vi "TPM and WF version 8-3.vi"() -> ()   [LabVIEW 2012]
uses:
  <vilib>/_Imagine Optic/VIs drivers/Data Haso/Wavefront parameters.ctl
  <vilib>/Utility/error.llb/DialogType.ctl
  Program Files/Imagine Optic/Casao LabVIEW SDK/Casao/Casao/Loop prefs.ctl
  <vilib>/_Imagine Optic/VIs drivers/Data Haso/DataHaso.ctl
  <vilib>/DAQmx/write.llb/DAQmx Write (Digital Bool 1Line 1Point).vi
  <vilib>/DAQmx/write.llb/DAQmx Write (Analog DBL 1Chan 1Samp).vi
  <vilib>/DAQmx/write.llb/DAQmx Write (Analog 1D Wfm NChan NSamp).vi
  <vilib>/DAQmx/create/channels.llb/DAQmx Create Channel (DO-Digital Output).vi
  <vilib>/DAQmx/create/channels.llb/DAQmx Create Channel (AO-Voltage-Basic).vi
  <vilib>/DAQmx/miscellaneous.llb/DAQmx Fill In Error Info.vi
  <vilib>/Analysis/coordinate.llb/2D Cartesian Coordinate Rotation (Array).vi
  <vilib>/DAQmx/configure/timing.llb/DAQmx Timing (Use Waveform).vi
  <vilib>/DAQmx/configure/trigger.llb/DAQmx Start Trigger (Digital Edge).vi
  <vilib>/measure/NI_MABase.lvlib
  <vilib>/Analysis/NI_AALPro.lvlib
panel:
  in  "Tab Control":enum32{"TPM imaging", "Wavefront sensor"}(tab)
  in  "Boolean 3":bool
  in  "Y offset (Pixel)":dbl=501.0
  in  "X offset (pixel)":dbl=502.0
  in  "Area Scale factor(0-1)":dbl=1.0
  in  "Model":i16(ring)=-5 items=["Phase"=1, "Imaging"=-5]
  out "Boolean":bool
  in  "Pockel Cell Correction Phase":dbl=135.0
  in  "Repeat time":dbl=100.0
  in  "Laser power %(0-100)":dbl=10.0
  in  "Exp Time":u32(ring)=500000 items=["0.5s"=500000, "1.0s"=1000000, "1.5s"=1500000]
  out "RMS 2":dbl
  out "PV 2":dbl
  in  "Filter x tilt 2":bool=TRUE
  in  "Filter y tilt 2":bool=TRUE
  in  "Curvature filter 2":bool=TRUE
  out "after correction":T1
  in  "Boolean 2":bool
  out "after correction":dbl[][](graph) caption="Wavefront"
  out "before correction":dbl[][](graph) caption="Wavefront"
  in  "Matrix path":path=path "C:/Documents and Settings/User/Desktop/zw/20160103 interaction matrix 1um bead step0.2.aomc"
  in  "Phase modulator config file path":path=path "C:/Program Files/Imagine Optic/Configuration Files/mirao 52-e 0225.xml"
  in  "Haso serial number":u32=7364
  in  "Scale factor":u16=1
  in  "Power%(0-100)":dbl=10.0
  in  "Filter x tilt":bool=TRUE
  in  "Filter y tilt":bool=TRUE
  in  "Curvature filter":bool=TRUE
  out "Parameters":T1
  out "Camera image":u32[][](graph)
  out "PV":dbl
  out "RMS":dbl
  # "For small area setting"
  # "Measure"
  # "Correction"
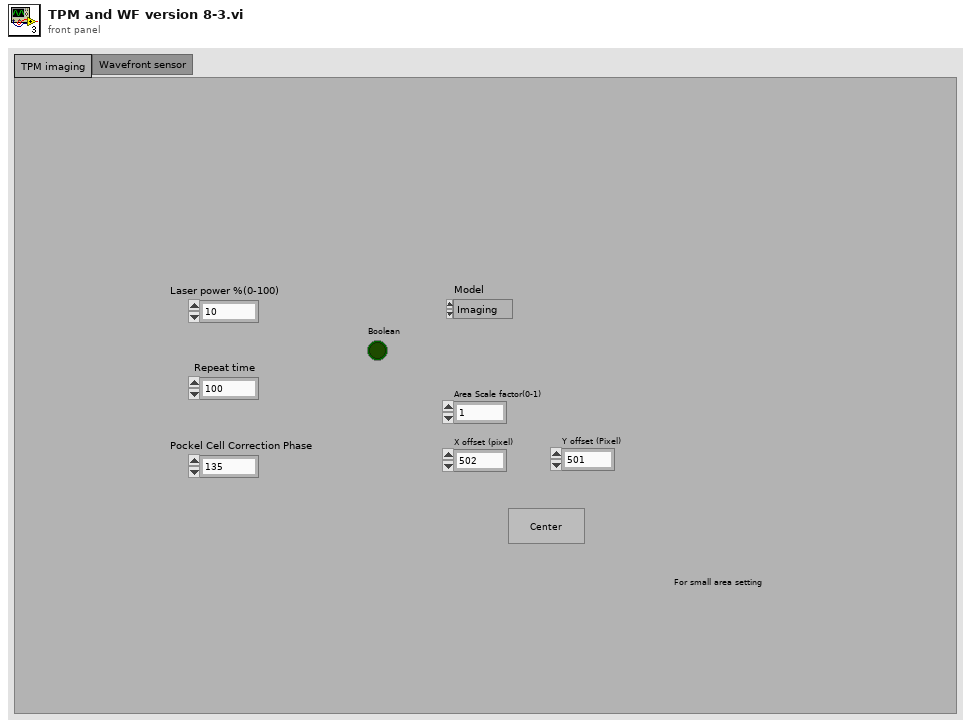
[diagram p1: front panel]
types:
  T1 = typedef "Wavefront parameters.ctl" = cluster{"X Tilt (mrad)":sgl, "Y Tilt (mrad)":sgl, "Radius of curvature (mm)":sgl, "X focal point position (mm)":sgl, "Y focal point position (mm)":sgl, "Astigmatism angle (rad)":sgl, "Sagittal focal length (mm)":sgl, "Tangential focal length (mm)":sgl}
  T2 = cluster{"Galvo/Pockels Cell Sampling Info":dbl, "#s":dbl}
  T3 = cluster{"Filtre tilt X":bool, "Filtre tilt Y":bool, "Filtre courbure":bool}
  T4 = typedef "Loop prefs.ctl" = cluster{"Filter tilt on measurement (closed loop)":bool, "Correction gain (closed loop)":sgl, "Limit of subapertures off in CGP (%)":sgl, "Limit of saturated actuators (%)":sgl}
  T5 = typedef "DataHaso.ctl" = i32
  T6 = cluster{"Measurement":T5, "Target":T5, "Manual target":T5}
  T7 = cluster{"Target for tilt":T5, "Target for focus":T5, "Target for all other aberrations":T5}
  T8 = typedef "DialogType.ctl" = u16
  T9 = typedef "Haso.ctl" = i32
  T10 = typedef "Camera.ctl" = i32
  T11 = typedef "Camera preferences.ctl" = cluster{"Exposure duration (µs)":u32, "Exposure duration specified (µs)":u32, "Number of summed images":u32, "Trigger type":enum16{"Internal", "TTL", "Software"}, "Trigger event":enum16{"falling", "rising"}, "Remove background image":bool, "Background image":T12, "Path to background image":string, "Auto exposure":bool, "Auto exposure target (%)":sgl, "Auto exposure tolerance (%)":sgl, "Timeout delay (ms)":u32, "Delay after trigger (µs)":i32}
  T12 = typedef "Image Compat.ctl" = cluster{"Signed/unsigned":bool, "Number of bits":T13, "Internal object id":i32, "Internal data id":i32}
  T13 = typedef "Data alignment enum.ctl" = enum16{"8", "16", "32"}
  T14 = typedef "Casao.ctl" = i32
  T15 = typedef "CasaoMatrix.ctl" = i32
  T16 = typedef "PhaseModul.ctl" = i32
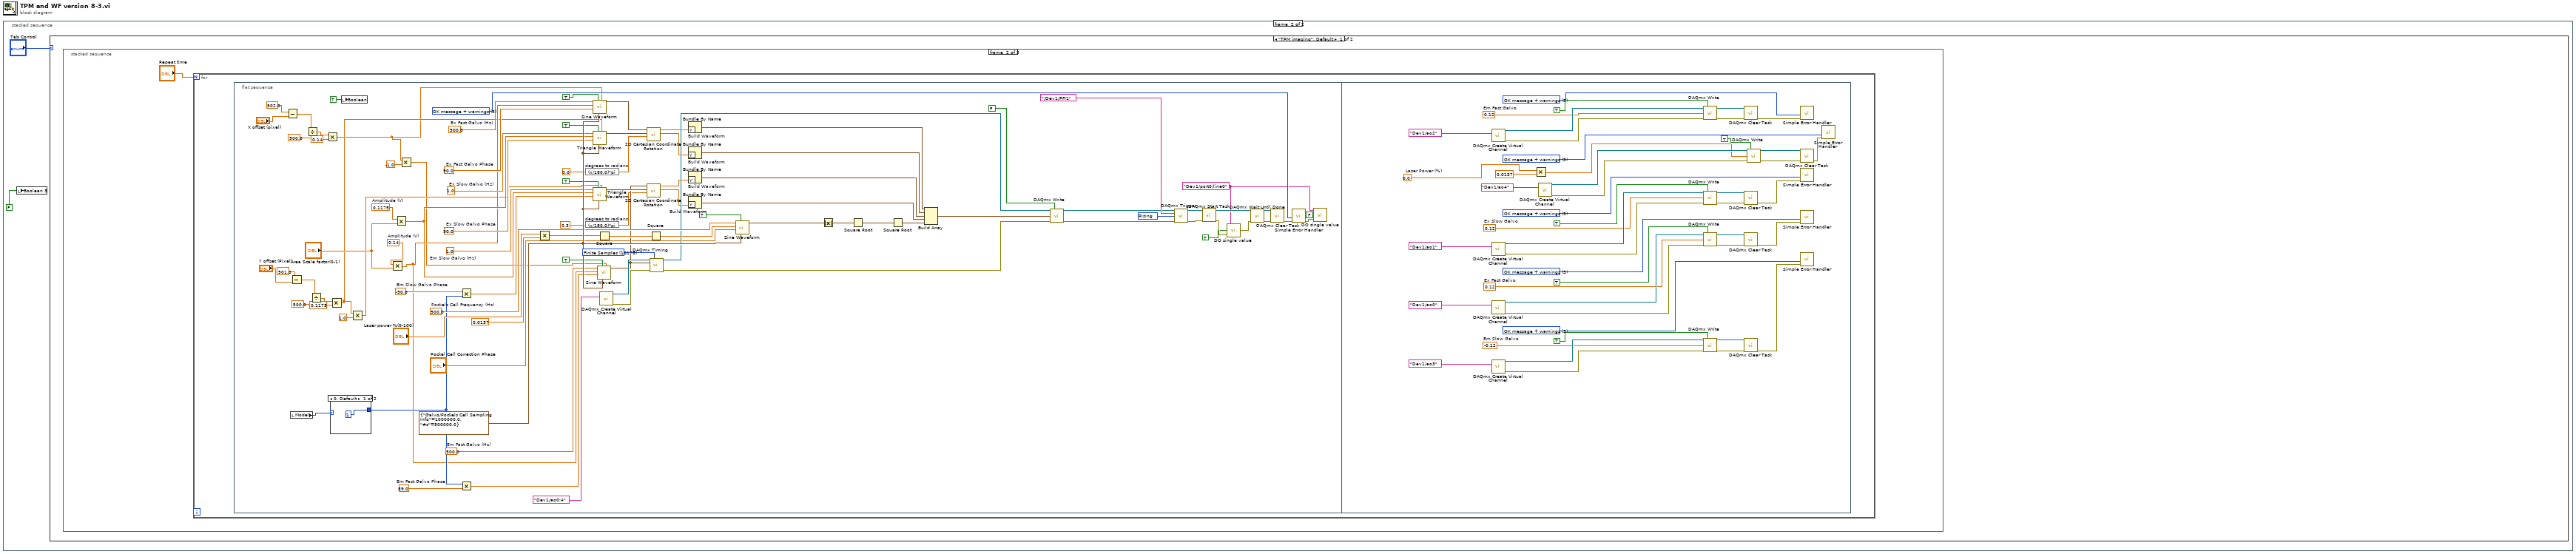
[diagram p0: block diagram]
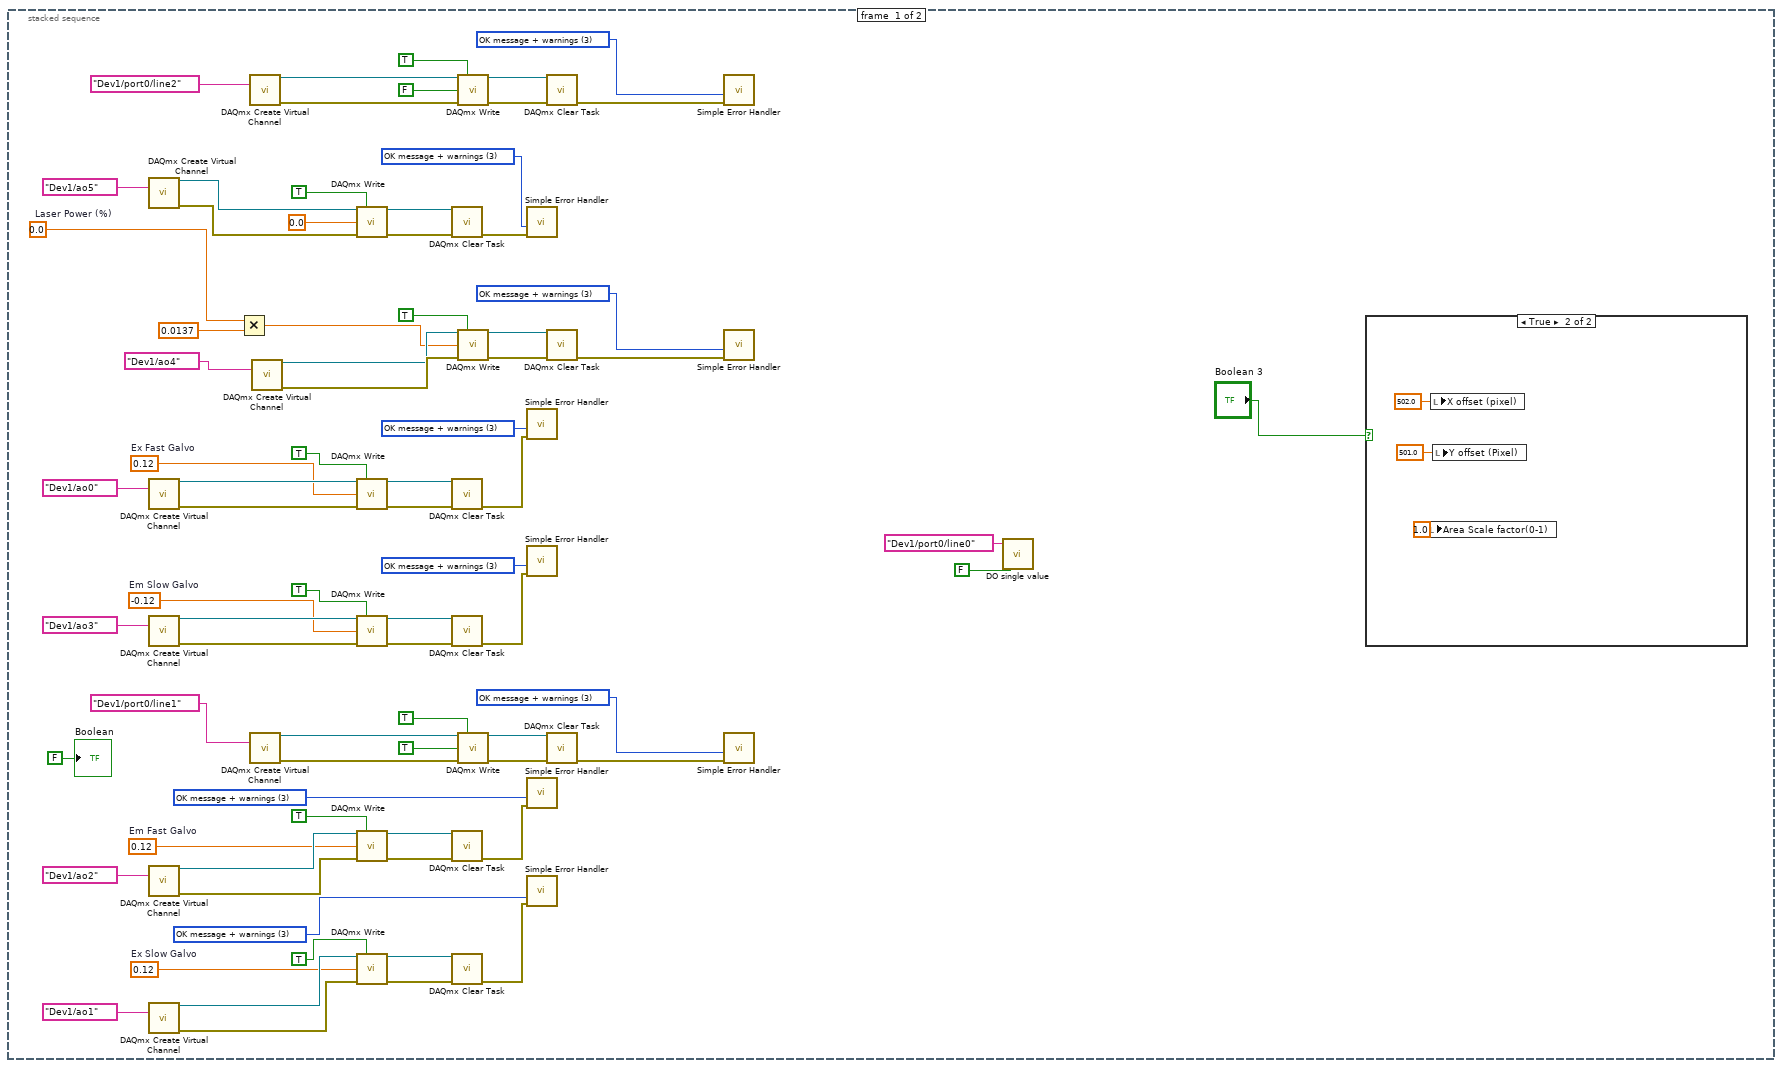
[diagram p2: hidden frame]
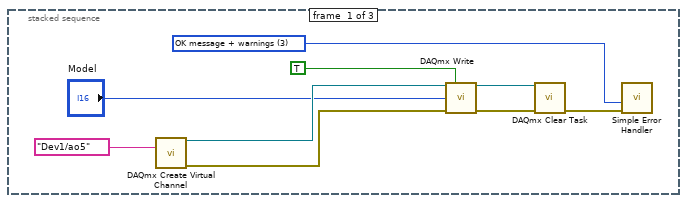
[diagram p4: hidden frame]
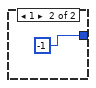
[diagram p5: hidden frame]
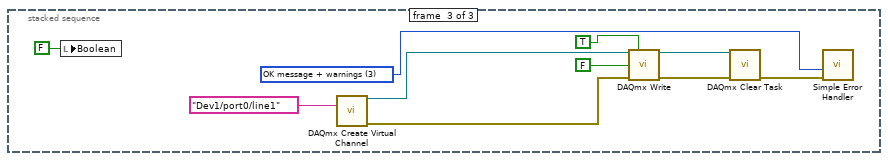
[diagram p6: hidden frame]
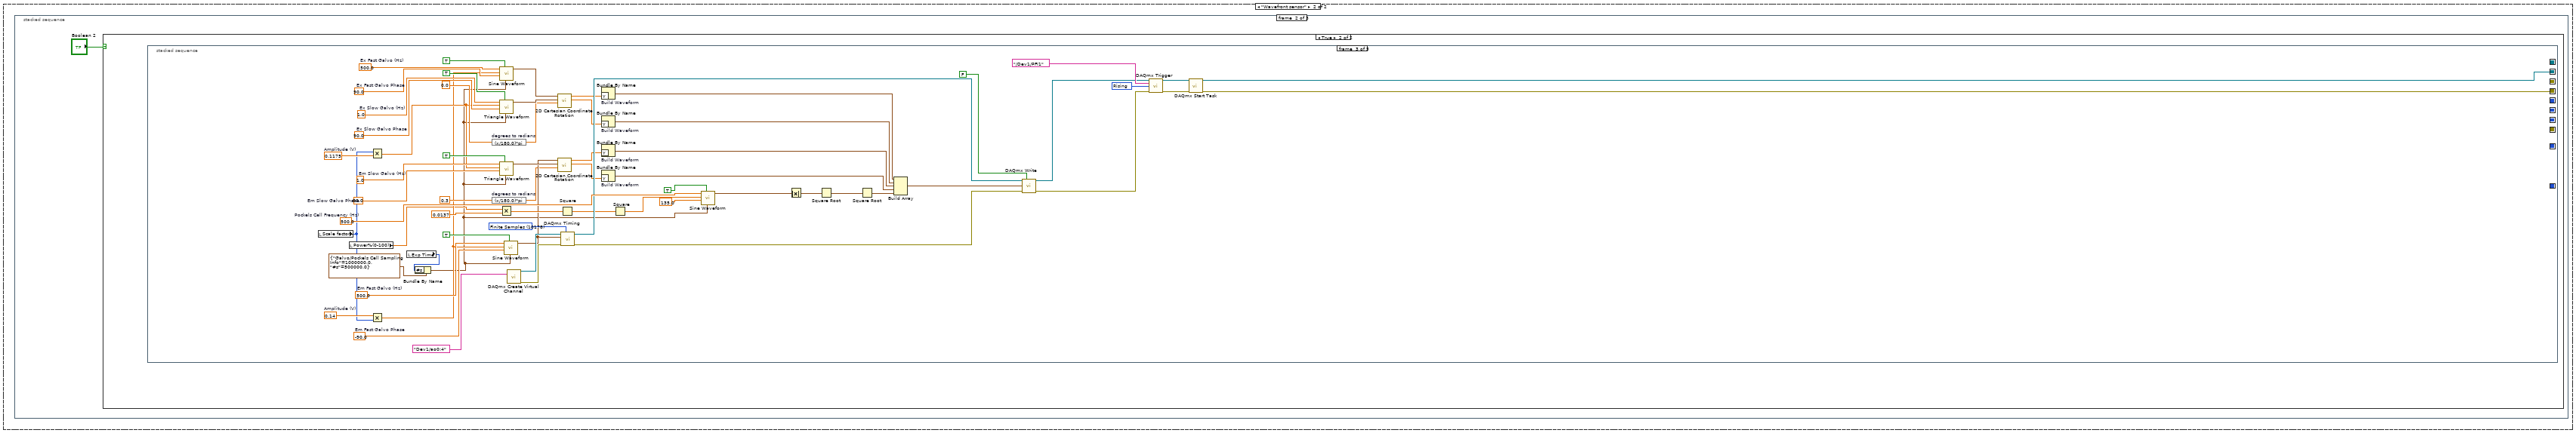
[diagram p7: hidden frame]
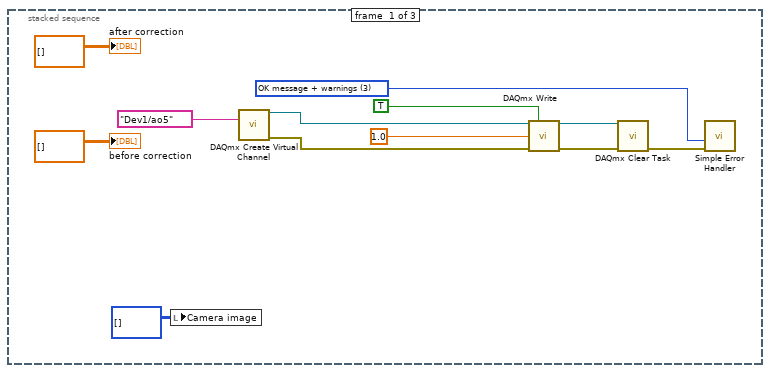
[diagram p8: hidden frame]
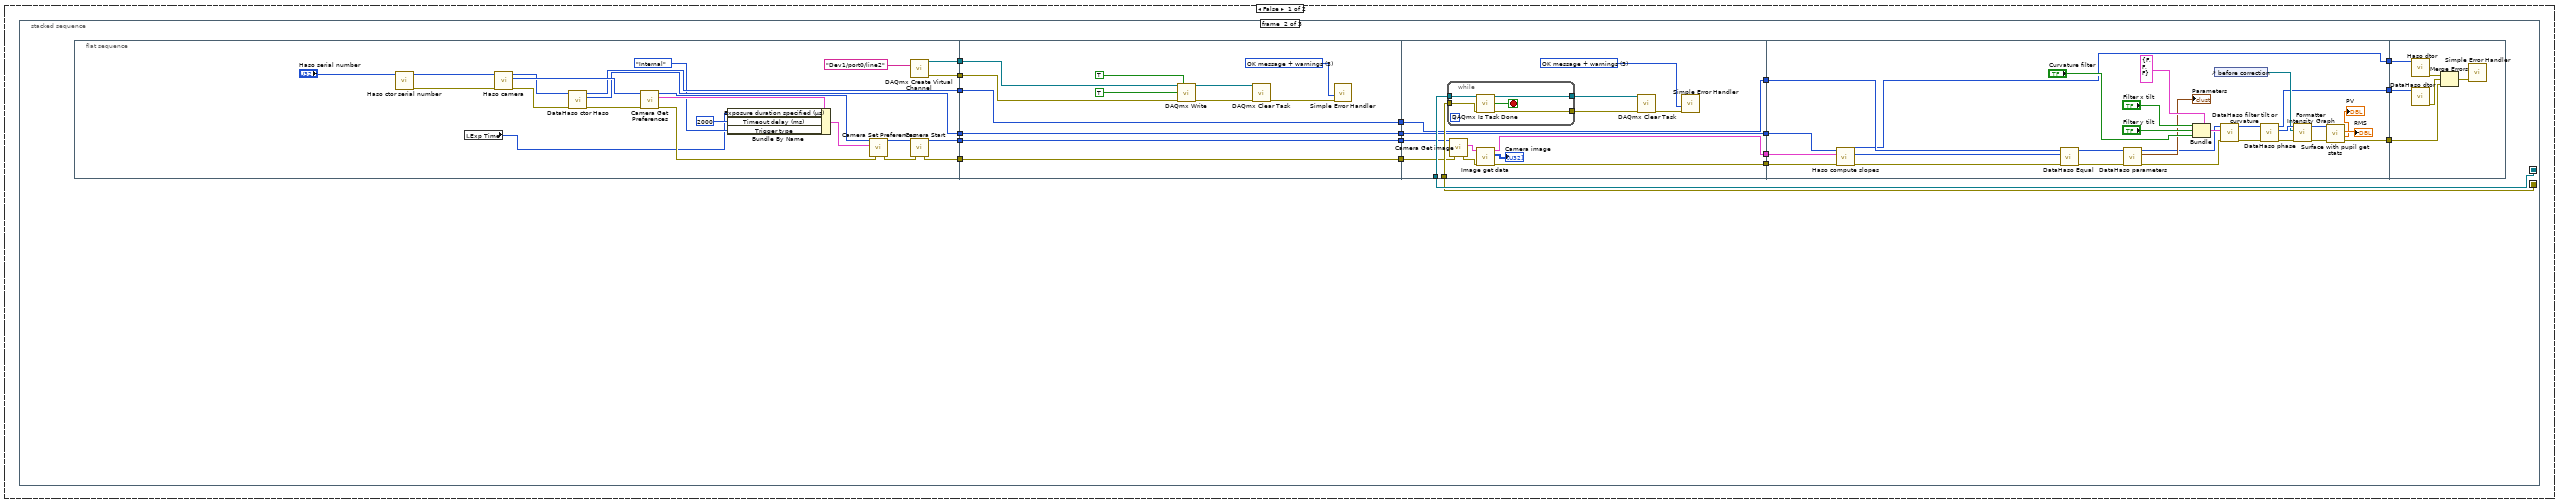
[diagram p9: hidden frame]
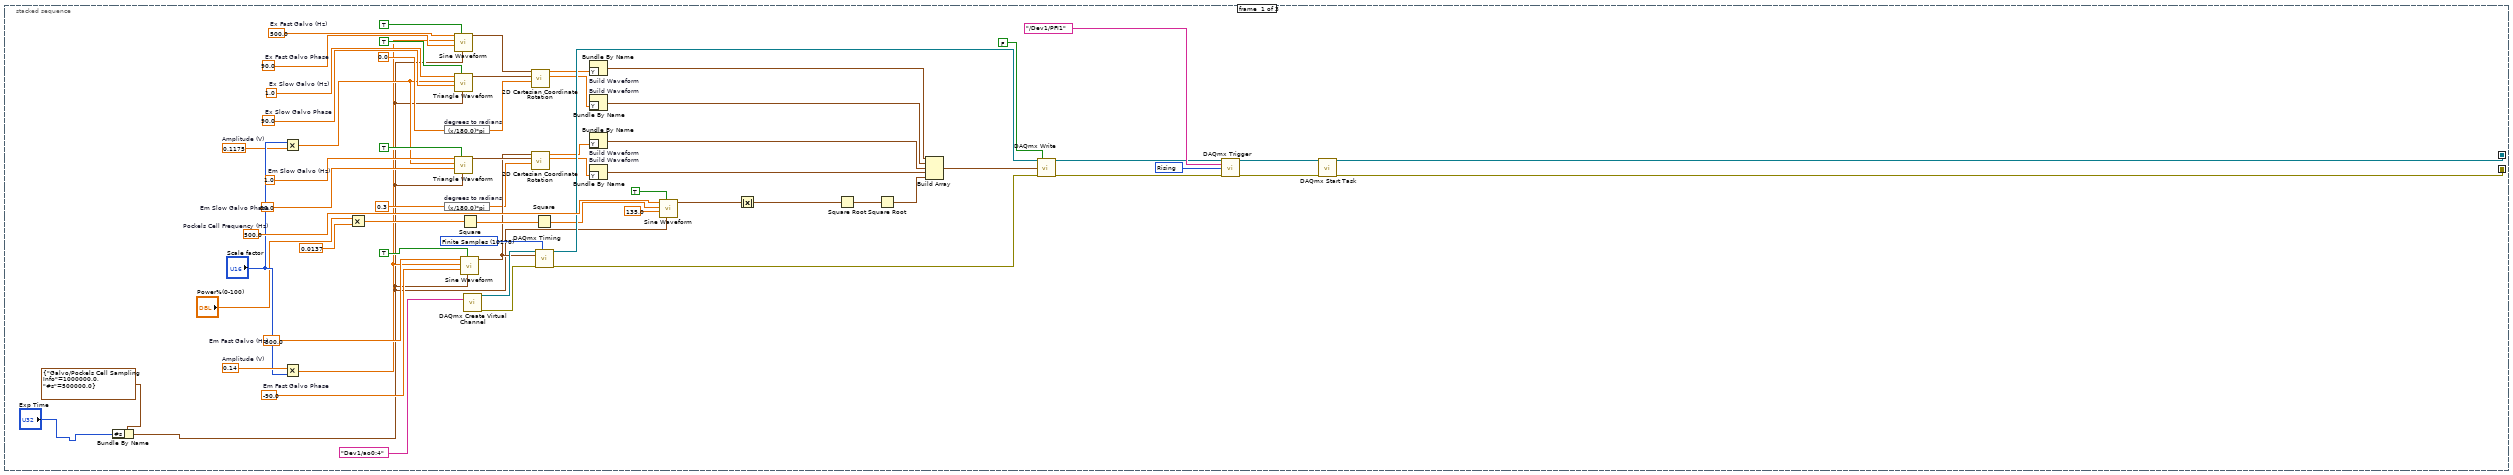
[diagram p10: hidden frame]
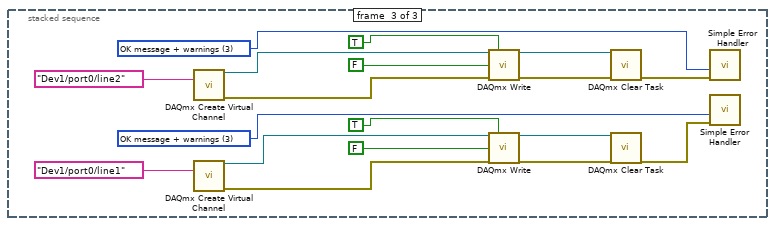
[diagram p11: hidden frame]
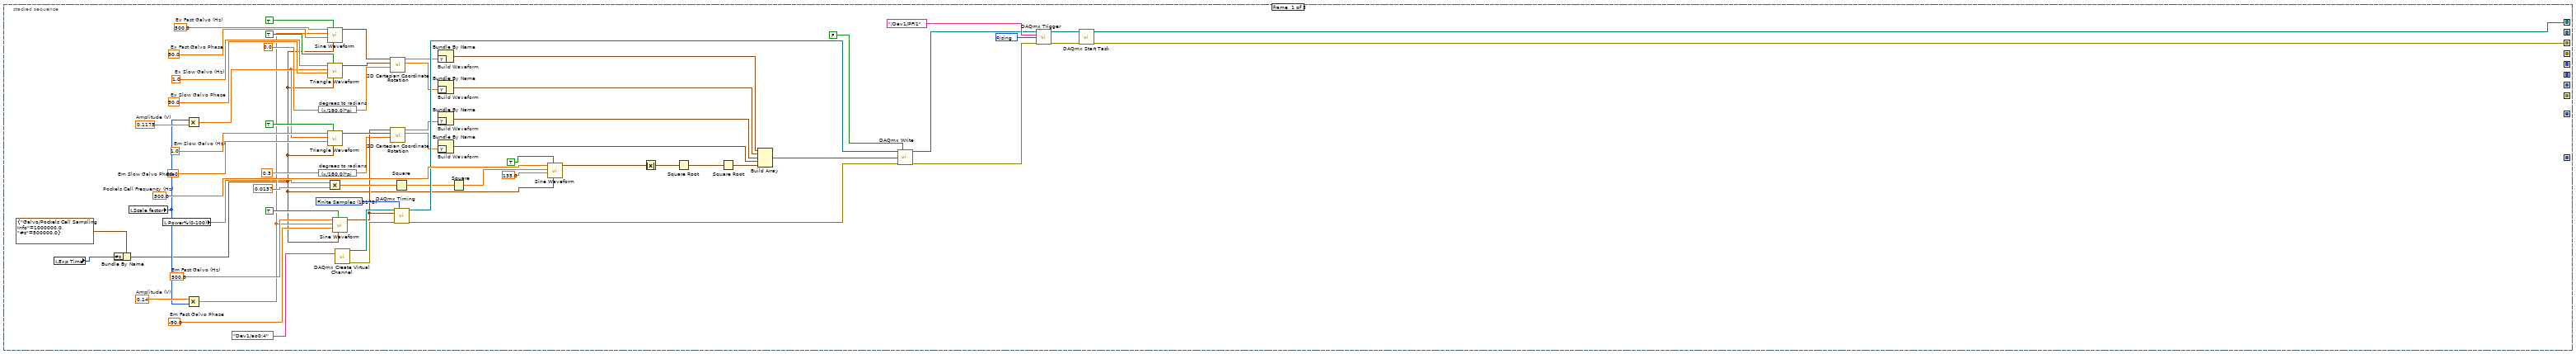
[diagram p12: hidden frame]
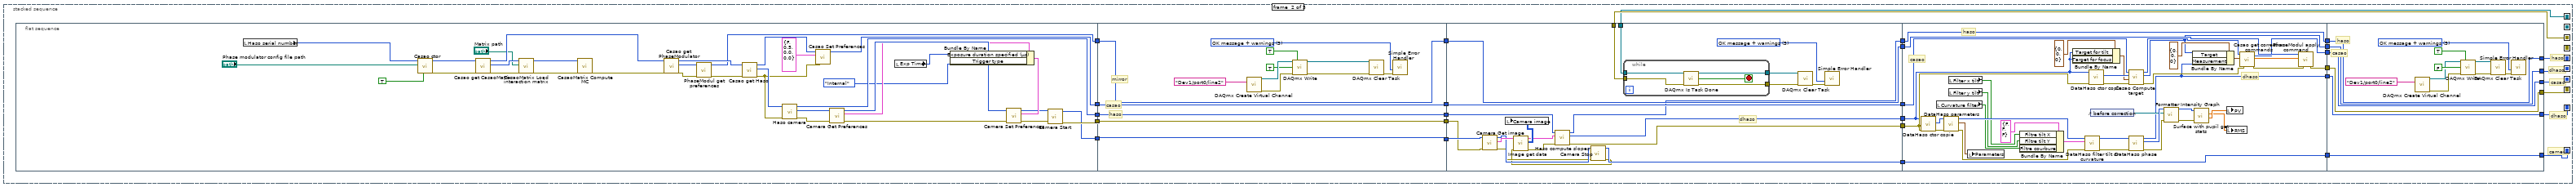
[diagram p13: hidden frame]
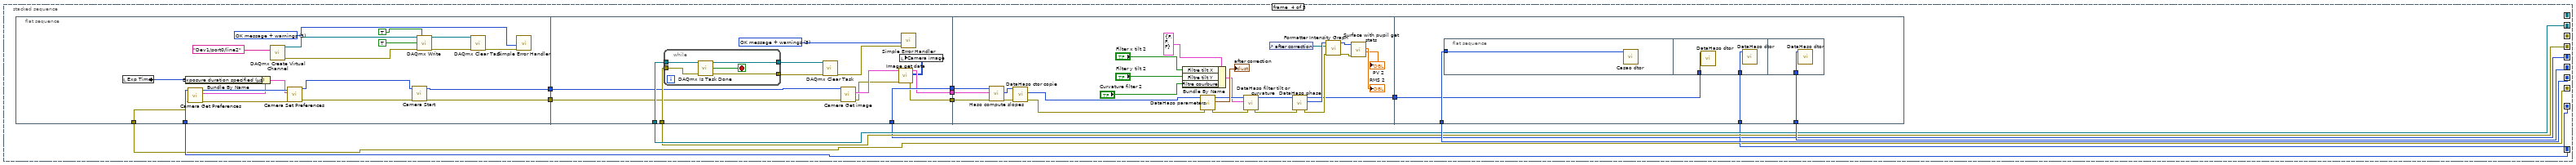
[diagram p14: hidden frame]
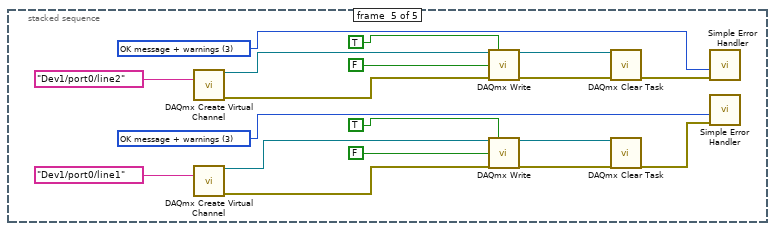
[diagram p15: hidden frame]
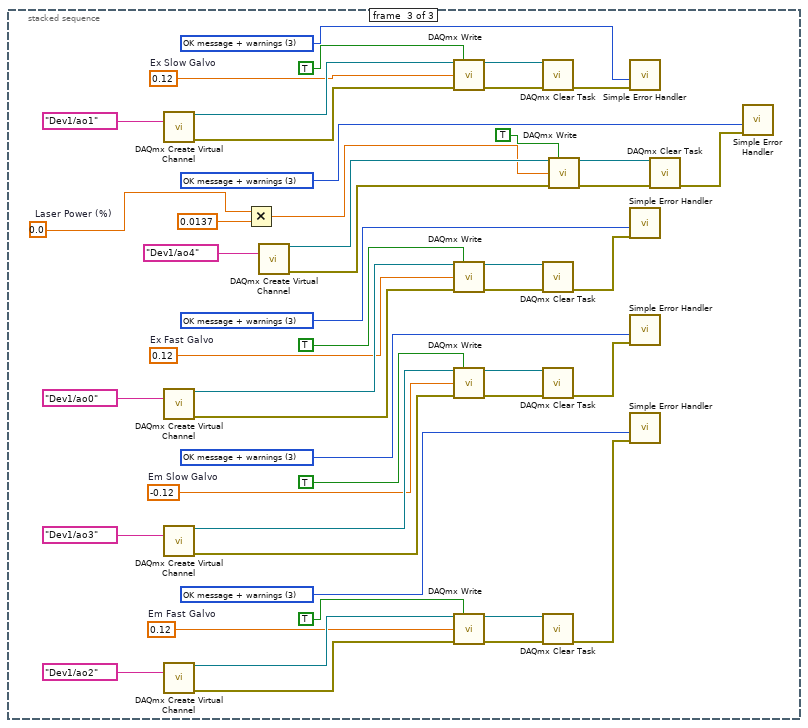
[diagram p16: hidden frame]
diagram:
  n1 = stacked-sequence {
    frame #0 {
      w11 = T8 3 items=["no dialog", "OK message", "continue or stop message", "OK message + warnings", "continue/stop + warnings"] ("type of dialog (OK msg:1)")
      w20 = T8 3 items=["no dialog", "OK message", "continue or stop message", "OK message + warnings", "continue/stop + warnings"] ("type of dialog (OK msg:1)")
      w59 = 0.0  # Laser Power (%)
      w41 = 0.12  # Em Fast Galvo
      w23 = -0.12  # Em Slow Galvo
      w32 = 0.12  # Ex Slow Galvo
      w50 = 0.12  # Ex Fast Galvo
      w29 = T8 3 items=["no dialog", "OK message", "continue or stop message", "OK message + warnings", "continue/stop + warnings"] ("type of dialog (OK msg:1)")
      w38 = T8 3 items=["no dialog", "OK message", "continue or stop message", "OK message + warnings", "continue/stop + warnings"] ("type of dialog (OK msg:1)")
      w47 = T8 3 items=["no dialog", "OK message", "continue or stop message", "OK message + warnings", "continue/stop + warnings"] ("type of dialog (OK msg:1)")
      w56 = T8 3 items=["no dialog", "OK message", "continue or stop message", "OK message + warnings", "continue/stop + warnings"] ("type of dialog (OK msg:1)")
      w62 = T8 3 items=["no dialog", "OK message", "continue or stop message", "OK message + warnings", "continue/stop + warnings"] ("type of dialog (OK msg:1)")
      w77 = T8 3 items=["no dialog", "OK message", "continue or stop message", "OK message + warnings", "continue/stop + warnings"] ("type of dialog (OK msg:1)")
      n2 = call-poly <vilib>:"DAQmx Create Virtual Channel.vi"("physical channels"=tag "Dev1/ao5") -> ("task out"=w16:refnum<k21>, "error out"=w15:errorcluster)  [unwired: 13 in]
      n3 = call-poly <vilib>:"DAQmx Create Virtual Channel.vi"("physical channels"=tag "Dev1/ao0") -> ("task out"=w52:refnum<k21>, "error out"=w51:errorcluster)  [unwired: 13 in]
      n4 = call-poly <vilib>:"DAQmx Create Virtual Channel.vi"("physical channels"=tag "Dev1/ao3") -> ("task out"=w25:refnum<k21>, "error out"=w24:errorcluster)  [unwired: 13 in]
      n5 = call-poly <vilib>:"DAQmx Create Virtual Channel.vi"("physical channels"=tag "Dev1/ao2") -> ("task out"=w43:refnum<k21>, "error out"=w42:errorcluster)  [unwired: 13 in]
      n6 = call-poly <vilib>:"DAQmx Create Virtual Channel.vi"("physical channels"=tag "Dev1/ao1") -> ("task out"=w34:refnum<k21>, "error out"=w33:errorcluster)  [unwired: 13 in]
      n7 = Multiply(x=w59, y=0.0137 ("data")) -> (x*y=w61:dbl)
      n8 = call-poly <vilib>:"DAQmx Create Virtual Channel.vi"("lines"=tag "Dev1/port0/line2") -> ("task out"=w7:refnum<k21>, "error out"=w8:errorcluster)  [unwired: 13 in]
      n9 = call-poly <vilib>:"DAQmx Create Virtual Channel.vi"("lines"=tag "Dev1/port0/line1") -> ("task out"=w73:refnum<k21>, "error out"=w74:errorcluster)  [unwired: 13 in]
      n10 = call-poly <vilib>:"DAQmx Create Virtual Channel.vi"("physical channels"=tag "Dev1/ao4") -> ("task out"=w68:refnum<k21>, "error out"=w69:errorcluster)  [unwired: 13 in]
      n11 = call-poly <vilib>:"DAQmx Write.vi"("task/channels in"=w16, "auto start"=TRUE, "data"=0.0, "error in"=w15) -> ("task out"=w18:refnum<k21>, "error out"=w17:errorcluster)  [unwired: 9 in, 1 out]
      n12 = call-poly <vilib>:"DAQmx Write.vi"("task/channels in"=w52, "auto start"=TRUE, "data"=w50, "error in"=w51) -> ("task out"=w54:refnum<k21>, "error out"=w53:errorcluster)  [unwired: 9 in, 1 out]
      n13 = call-poly <vilib>:"DAQmx Write.vi"("task/channels in"=w25, "auto start"=TRUE, "data"=w23, "error in"=w24) -> ("task out"=w27:refnum<k21>, "error out"=w26:errorcluster)  [unwired: 9 in, 1 out]
      n14 = call-poly <vilib>:"DAQmx Write.vi"("task/channels in"=w43, "auto start"=TRUE, "data"=w41, "error in"=w42) -> ("task out"=w45:refnum<k21>, "error out"=w44:errorcluster)  [unwired: 9 in, 1 out]
      n15 = call-poly <vilib>:"DAQmx Write.vi"("task/channels in"=w34, "auto start"=TRUE, "data"=w32, "error in"=w33) -> ("task out"=w36:refnum<k21>, "error out"=w35:errorcluster)  [unwired: 9 in, 1 out]
      n16 = call <vilib>:"DAQmx Clear Task.vi"("task in"=w18, "error in"=w17) -> ("error out"=w19:errorcluster)  [unwired: 13 in]
      n17 = call <vilib>:"DAQmx Clear Task.vi"("task in"=w54, "error in"=w53) -> ("error out"=w55:errorcluster)  [unwired: 13 in]
      n18 = call <vilib>:"DAQmx Clear Task.vi"("task in"=w27, "error in"=w26) -> ("error out"=w28:errorcluster)  [unwired: 13 in]
      n19 = call <vilib>:"DAQmx Clear Task.vi"("task in"=w45, "error in"=w44) -> ("error out"=w46:errorcluster)  [unwired: 13 in]
      n20 = call <vilib>:"DAQmx Clear Task.vi"("task in"=w36, "error in"=w35) -> ("error out"=w37:errorcluster)  [unwired: 13 in]
      n21 = call-poly <vilib>:"DAQmx Write.vi"("task/channels in"=w7, "auto start"=TRUE, "data"=FALSE ("Shutter"), "error in"=w8) -> ("task out"=w5:refnum<k21>, "error out"=w4:errorcluster)  [unwired: 9 in, 1 out]
      n22 = call-poly <vilib>:"DAQmx Write.vi"("task/channels in"=w68, "auto start"=TRUE, "data"=w61, "error in"=w69) -> ("task out"=w65:refnum<k21>, "error out"=w66:errorcluster)  [unwired: 9 in, 1 out]
      n23 = call-poly <vilib>:"DAQmx Write.vi"("task/channels in"=w73, "auto start"=TRUE, "data"=TRUE ("Shutter"), "error in"=w74) -> ("task out"=w71:refnum<k21>, "error out"=w70:errorcluster)  [unwired: 9 in, 1 out]
      n24 = call <vilib>:"Simple Error Handler.vi"("type of dialog (OK msg:1)"=w20, "error in (no error)"=w19) -> ()  [unwired: 3 in, 5 out]
      n25 = call <vilib>:"Simple Error Handler.vi"("type of dialog (OK msg:1)"=w56, "error in (no error)"=w55) -> ()  [unwired: 3 in, 5 out]
      n26 = call <vilib>:"Simple Error Handler.vi"("type of dialog (OK msg:1)"=w29, "error in (no error)"=w28) -> ()  [unwired: 3 in, 5 out]
      n27 = call <vilib>:"Simple Error Handler.vi"("type of dialog (OK msg:1)"=w47, "error in (no error)"=w46) -> ()  [unwired: 3 in, 5 out]
      n28 = call <vilib>:"Simple Error Handler.vi"("type of dialog (OK msg:1)"=w38, "error in (no error)"=w37) -> ()  [unwired: 3 in, 5 out]
      n29 = call <vilib>:"DAQmx Clear Task.vi"("task in"=w5, "error in"=w4) -> ("error out"=w10:errorcluster)  [unwired: 13 in]
      n30 = call <vilib>:"DAQmx Clear Task.vi"("task in"=w65, "error in"=w66) -> ("error out"=w63:errorcluster)  [unwired: 13 in]
      n31 = call <vilib>:"DAQmx Clear Task.vi"("task in"=w71, "error in"=w70) -> ("error out"=w76:errorcluster)  [unwired: 13 in]
      n32 = call <vilib>:"Simple Error Handler.vi"("type of dialog (OK msg:1)"=w11, "error in (no error)"=w10) -> ()  [unwired: 3 in, 5 out]
      n33 = call <vilib>:"Simple Error Handler.vi"("type of dialog (OK msg:1)"=w62, "error in (no error)"=w63) -> ()  [unwired: 3 in, 5 out]
      n34 = call <vilib>:"Simple Error Handler.vi"("type of dialog (OK msg:1)"=w77, "error in (no error)"=w76) -> ()  [unwired: 3 in, 5 out]
      n35 = call "DO single value.vi"("data"=FALSE, "lines"=tag "Dev1/port0/line0") -> ()  [unwired: 1 in, 1 out]
      n36 = case shown="True" "Boolean 3" {
        frame False {
        }
        frame True {
          n37 = local write "Area Scale factor(0-1)"(1.0 ("Scale factor(0-1)")) -> ()
          n38 = local write "X offset (pixel)"(502.0 ("X offset (pixel)")) -> ()
          n39 = local write "Y offset (Pixel)"(501.0 ("Y offset (Pixel)")) -> ()
        }
      }
      "Boolean" <- FALSE ("Boolean")
    }
    frame #1 {
      n40 = local write "Boolean 3"(FALSE ("Boolean 3")) -> ()
      n41 = case shown="\"TPM imaging\", Default" "Tab Control" {
        frame "TPM imaging", Default {
          n42 = stacked-sequence {
            frame #0 {
              w87 = T8 3 items=["no dialog", "OK message", "continue or stop message", "OK message + warnings", "continue/stop + warnings"] ("type of dialog (OK msg:1)")
              n43 = call-poly <vilib>:"DAQmx Create Virtual Channel.vi"("physical channels"=tag "Dev1/ao5") -> ("task out"=w91:refnum<k21>, "error out"=w92:errorcluster)  [unwired: 13 in]
              n44 = call-poly <vilib>:"DAQmx Write.vi"("task/channels in"=w91, "auto start"=TRUE, "data"="Model", "error in"=w92) -> ("task out"=w89:refnum<k21>, "error out"=w90:errorcluster)  [unwired: 9 in, 1 out]
              n45 = call <vilib>:"DAQmx Clear Task.vi"("task in"=w89, "error in"=w90) -> ("error out"=w88:errorcluster)  [unwired: 13 in]
              n46 = call <vilib>:"Simple Error Handler.vi"("type of dialog (OK msg:1)"=w87, "error in (no error)"=w88) -> ()  [unwired: 3 in, 5 out]
            }
            frame #1 {
              n47 = for {
                N: "Repeat time" -> [_]
                n48 = flat-sequence {
                  frame #0 {
                    w118 = tag "Dev1/port0/line0" ("lines")
                    w129 = 89.0  # Em Fast Galvo Phase
                    w186 = 1.0  # Em Slow Galvo (Hz)
                    w184 = 1.0  # Ex Slow Galvo (Hz)
                    w116 = 0.1175  # Amplitude (V)
                    w183 = 500.0  # Ex Fast Galvo (Hz)
                    w113 = 0.14  # Amplitude (V)
                    w182 = 500.0  # Pockels Cell Frequency (Hz)
                    w187 = T2 {"Galvo/Pockels Cell Sampling Info"=1000000.0, "#s"=500000.0} ("Sampling Info")
                    w180 = 500.0  # Em Fast Galvo (Hz)
                    w131 = -90.0  # Em Slow Galvo Phase
                    w176 = 90.0  # Ex Slow Galvo Phase
                    w177 = 90.0  # Ex Fast Galvo Phase
                    w172 = T8 3 items=["no dialog", "OK message", "continue or stop message", "OK message + warnings", "continue/stop + warnings"] ("type of dialog (OK msg:1)")
                    w171 = 10280 items=["Rising"=10280, "Falling"=10171] ("edge")
                    w166 = 10178 items=["Finite Samples"=10178, "Continuous Samples"=10123, "Hardware Timed Single Point"=12522] ("sample mode")
                    n49 = Subtract(x=502.0 ("y"), y="X offset (pixel)") -> (x-y=w108:dbl)
                    n50 = Subtract(x=501.0 ("y"), y="Y offset (Pixel)") -> (x-y=w104:dbl)
                    n51 = local read "Model"() -> (w124:i16)
                    n52 = Divide(x=w108, y=500.0) -> (x/y=w110:dbl)
                    n53 = Divide(x=w104, y=500.0) -> (x/y=w106:dbl)
                    n54 = Multiply(x=w110, y=0.14) -> (x*y=w95:dbl)
                    n55 = Multiply(x=w106, y=0.1175) -> (x*y=w98:dbl)
                    n56 = case shown="0, Default" w124 {
                      tunnel: [1 -1] -> w123
                      frame 0, Default {
                      }
                      frame 1 {
                      }
                    }
                    n57 = local write "Boolean"(TRUE ("Boolean")) -> ()
                    n58 = Multiply(x=w98, y=1.0) -> (x*y=w97:dbl)
                    n59 = Multiply(x=w113, y="Area Scale factor(0-1)") -> (x*y=w112:dbl)
                    n60 = Multiply(x=w116, y="Area Scale factor(0-1)") -> (x*y=w115:dbl)
                    n61 = Multiply(x=w95, y=-1.0) -> (x*y=w94:dbl)
                    n62 = Multiply(x=w131, y=w123) -> (x*y=w130:dbl)
                    n63 = Multiply(x=w123, y=w129) -> (x*y=w128:dbl)
                    n64 = Multiply(x="Laser power %(0-100)", y=0.0137 ("data")) -> (x*y=w181:dbl)
                    n65 = expression code="(x/180.0)*pi" "degrees to radians"(0.0 ("Ex Theta")) -> (w138:dbl)
                    n66 = expression code="(x/180.0)*pi" "degrees to radians"(0.3 ("Em Theta")) -> (w135:dbl)
                    n67 = call <vilib>:"Sine Waveform.vi"("offset"=w95, "sampling info"=w187, "reset signal"=TRUE, "phase"=w177, "amplitude"=w112, "frequency"=w183) -> ("signal out"=w150:waveform(dbl))  [unwired: 4 in, 1 out]
                    n68 = call <vilib>:"Triangle Waveform.vi"("offset"=w98, "sampling info"=w187, "reset signal"=TRUE, "phase"=w176, "amplitude"=w115, "frequency"=w184) -> ("signal out"=w151:waveform(dbl))  [unwired: 4 in, 1 out]
                    n69 = call <vilib>:"Triangle Waveform.vi"("offset"=w97, "sampling info"=w187, "reset signal"=TRUE, "phase"=w130, "amplitude"=w115, "frequency"=w186) -> ("signal out"=w142:waveform(dbl))  [unwired: 4 in, 1 out]
                    n70 = call <vilib>:"Sine Waveform.vi"("offset"=w94, "sampling info"=w187, "reset signal"=TRUE, "phase"=w128, "amplitude"=w112, "frequency"=w180) -> ("signal out"=w137:waveform(dbl))  [unwired: 4 in, 1 out]
                    n71 = Square(x=w181) -> (x^2=w153:dbl)
                    n72 = call-poly <vilib>:"DAQmx Create Virtual Channel.vi"("physical channels"=tag "Dev1/ao0:4") -> ("task out"=w168:refnum<k21>, "error out"=w161:errorcluster)  [unwired: 13 in]
                    n73 = call-poly <vilib>:"2D Cartesian Coordinate Rotation.vi"("theta"=w138, "Y"=w151, "X"=w150) -> ("Y Out"=w147:dbl[], "X Out"=w149:dbl[])  [unwired: 6 in, 1 out]
                    n74 = call-poly <vilib>:"2D Cartesian Coordinate Rotation.vi"("theta"=w135, "Y"=w142, "X"=w137) -> ("Y Out"=w143:dbl[], "X Out"=w144:dbl[])  [unwired: 6 in, 1 out]
                    n75 = Square(x=w153) -> (x^2=w152:dbl)
                    n76 = call-poly <vilib>:"DAQmx Timing.vi"("task/channels in"=w168, "sample mode"=w166, "waveform"=w137, "error in"=w161) -> ("task out"=w162:refnum<k21>, "error out"=w163:errorcluster)  [unwired: 10 in]
                    n77 = Bundle By Name "Build Waveform"("Y"=w149) -> (w148:waveform(dbl))  [unwired: 1 in]
                    n78 = Bundle By Name "Build Waveform"("Y"=w147) -> (w146:waveform(dbl))  [unwired: 1 in]
                    n79 = Bundle By Name "Build Waveform"("Y"=w144) -> (w140:waveform(dbl))  [unwired: 1 in]
                    n80 = Bundle By Name "Build Waveform"("Y"=w143) -> (w141:waveform(dbl))  [unwired: 1 in]
                    n81 = call <vilib>:"Sine Waveform.vi"("sampling info"=w187, "reset signal"=TRUE, "phase"="Pockel Cell Correction Phase", "amplitude"=w152, "frequency"=w182) -> ("signal out"=w179:waveform(dbl))  [unwired: 5 in, 1 out]
                    n82 = Absolute Value(x=w179) -> (abs(x)=w155:waveform(dbl))
                    n83 = Square Root(x=w155) -> (sqrt(x)=w154:waveform(dbl))
                    n84 = Square Root(x=w154) -> (sqrt(x)=w145:waveform(dbl))
                    n85 = Build Array "Build Array"(w148, w146, w140, w141, w145) -> (w169:waveform(dbl)[])
                    n86 = call-poly <vilib>:"DAQmx Write.vi"("task/channels in"=w162, "auto start"=FALSE, "data"=w169, "error in"=w163) -> ("task out"=w164:refnum<k21>, "error out"=w165:errorcluster)  [unwired: 9 in, 1 out]
                    n87 = call-poly <vilib>:"DAQmx Trigger.vi"("task/channels in"=w164, "source"=tag "/Dev1/PFI1", "edge"=w171, "error in"=w165) -> ("task out"=w174:refnum<k21>, "error out"=w175:errorcluster)  [unwired: 10 in]
                    n88 = call <vilib>:"DAQmx Start Task.vi"("task/channels in"=w174, "error in"=w175) -> ("task out"=w127:refnum<k21>, "error out"=w122:errorcluster)  [unwired: 12 in]
                    n89 = call "DO single value.vi"("error in"=w122, "data"=TRUE, "lines"=w118) -> ("error out"=w121:errorcluster)
                    n90 = call <vilib>:"DAQmx Wait Until Done.vi"("task/channels in"=w127, "error in"=w121) -> ("task out"=w126:refnum<k21>, "error out"=w125:errorcluster)  [unwired: 12 in]
                    n91 = call <vilib>:"DAQmx Clear Task.vi"("task in"=w126, "error in"=w125) -> ("error out"=w173:errorcluster)  [unwired: 13 in]
                    n92 = call <vilib>:"Simple Error Handler.vi"("type of dialog (OK msg:1)"=w172, "error in (no error)"=w173) -> ("error out"=w119:errorcluster)  [unwired: 3 in, 4 out]
                    n93 = call "DO single value.vi"("error in"=w119, "data"=FALSE, "lines"=w118) -> ()  [unwired: 1 out]
                  }
                  frame #1 {
                    w226 = 0.0  # Laser Power (%)
                    w208 = 0.12  # Em Fast Galvo
                    w190 = -0.12  # Em Slow Galvo
                    w199 = 0.12  # Ex Slow Galvo
                    w217 = 0.12  # Ex Fast Galvo
                    w196 = T8 3 items=["no dialog", "OK message", "continue or stop message", "OK message + warnings", "continue/stop + warnings"] ("type of dialog (OK msg:1)")
                    w205 = T8 3 items=["no dialog", "OK message", "continue or stop message", "OK message + warnings", "continue/stop + warnings"] ("type of dialog (OK msg:1)")
                    w214 = T8 3 items=["no dialog", "OK message", "continue or stop message", "OK message + warnings", "continue/stop + warnings"] ("type of dialog (OK msg:1)")
                    w223 = T8 3 items=["no dialog", "OK message", "continue or stop message", "OK message + warnings", "continue/stop + warnings"] ("type of dialog (OK msg:1)")
                    w229 = T8 3 items=["no dialog", "OK message", "continue or stop message", "OK message + warnings", "continue/stop + warnings"] ("type of dialog (OK msg:1)")
                    n94 = call-poly <vilib>:"DAQmx Create Virtual Channel.vi"("physical channels"=tag "Dev1/ao2") -> ("task out"=w210:refnum<k21>, "error out"=w209:errorcluster)  [unwired: 13 in]
                    n95 = call-poly <vilib>:"DAQmx Create Virtual Channel.vi"("physical channels"=tag "Dev1/ao1") -> ("task out"=w201:refnum<k21>, "error out"=w200:errorcluster)  [unwired: 13 in]
                    n96 = call-poly <vilib>:"DAQmx Create Virtual Channel.vi"("physical channels"=tag "Dev1/ao0") -> ("task out"=w219:refnum<k21>, "error out"=w218:errorcluster)  [unwired: 13 in]
                    n97 = call-poly <vilib>:"DAQmx Create Virtual Channel.vi"("physical channels"=tag "Dev1/ao3") -> ("task out"=w192:refnum<k21>, "error out"=w191:errorcluster)  [unwired: 13 in]
                    n98 = Multiply(x=w226, y=0.0137 ("data")) -> (x*y=w228:dbl)
                    n99 = call-poly <vilib>:"DAQmx Create Virtual Channel.vi"("physical channels"=tag "Dev1/ao4") -> ("task out"=w235:refnum<k21>, "error out"=w236:errorcluster)  [unwired: 13 in]
                    n100 = call-poly <vilib>:"DAQmx Write.vi"("task/channels in"=w210, "auto start"=TRUE, "data"=w208, "error in"=w209) -> ("task out"=w212:refnum<k21>, "error out"=w211:errorcluster)  [unwired: 9 in, 1 out]
                    n101 = call-poly <vilib>:"DAQmx Write.vi"("task/channels in"=w201, "auto start"=TRUE, "data"=w199, "error in"=w200) -> ("task out"=w203:refnum<k21>, "error out"=w202:errorcluster)  [unwired: 9 in, 1 out]
                    n102 = call-poly <vilib>:"DAQmx Write.vi"("task/channels in"=w219, "auto start"=TRUE, "data"=w217, "error in"=w218) -> ("task out"=w221:refnum<k21>, "error out"=w220:errorcluster)  [unwired: 9 in, 1 out]
                    n103 = call-poly <vilib>:"DAQmx Write.vi"("task/channels in"=w192, "auto start"=TRUE, "data"=w190, "error in"=w191) -> ("task out"=w194:refnum<k21>, "error out"=w193:errorcluster)  [unwired: 9 in, 1 out]
                    n104 = call <vilib>:"DAQmx Clear Task.vi"("task in"=w212, "error in"=w211) -> ("error out"=w213:errorcluster)  [unwired: 13 in]
                    n105 = call <vilib>:"DAQmx Clear Task.vi"("task in"=w203, "error in"=w202) -> ("error out"=w204:errorcluster)  [unwired: 13 in]
                    n106 = call <vilib>:"DAQmx Clear Task.vi"("task in"=w221, "error in"=w220) -> ("error out"=w222:errorcluster)  [unwired: 13 in]
                    n107 = call <vilib>:"DAQmx Clear Task.vi"("task in"=w194, "error in"=w193) -> ("error out"=w195:errorcluster)  [unwired: 13 in]
                    n108 = call-poly <vilib>:"DAQmx Write.vi"("task/channels in"=w235, "auto start"=TRUE, "data"=w228, "error in"=w236) -> ("task out"=w232:refnum<k21>, "error out"=w233:errorcluster)  [unwired: 9 in, 1 out]
                    n109 = call <vilib>:"Simple Error Handler.vi"("type of dialog (OK msg:1)"=w214, "error in (no error)"=w213) -> ()  [unwired: 3 in, 5 out]
                    n110 = call <vilib>:"DAQmx Clear Task.vi"("task in"=w232, "error in"=w233) -> ("error out"=w230:errorcluster)  [unwired: 13 in]
                    n111 = call <vilib>:"Simple Error Handler.vi"("type of dialog (OK msg:1)"=w205, "error in (no error)"=w204) -> ()  [unwired: 3 in, 5 out]
                    n112 = call <vilib>:"Simple Error Handler.vi"("type of dialog (OK msg:1)"=w223, "error in (no error)"=w222) -> ()  [unwired: 3 in, 5 out]
                    n113 = call <vilib>:"Simple Error Handler.vi"("type of dialog (OK msg:1)"=w196, "error in (no error)"=w195) -> ()  [unwired: 3 in, 5 out]
                    n114 = call <vilib>:"Simple Error Handler.vi"("type of dialog (OK msg:1)"=w229, "error in (no error)"=w230) -> ()  [unwired: 3 in, 5 out]
                  }
                }
              }
            }
            frame #2 {
              w244 = T8 3 items=["no dialog", "OK message", "continue or stop message", "OK message + warnings", "continue/stop + warnings"] ("type of dialog (OK msg:1)")
              n115 = local write "Boolean"(FALSE ("Boolean")) -> ()
              n116 = call-poly <vilib>:"DAQmx Create Virtual Channel.vi"("lines"=tag "Dev1/port0/line1") -> ("task out"=w240:refnum<k21>, "error out"=w241:errorcluster)  [unwired: 13 in]
              n117 = call-poly <vilib>:"DAQmx Write.vi"("task/channels in"=w240, "auto start"=TRUE, "data"=FALSE ("Shutter"), "error in"=w241) -> ("task out"=w238:refnum<k21>, "error out"=w237:errorcluster)  [unwired: 9 in, 1 out]
              n118 = call <vilib>:"DAQmx Clear Task.vi"("task in"=w238, "error in"=w237) -> ("error out"=w243:errorcluster)  [unwired: 13 in]
              n119 = call <vilib>:"Simple Error Handler.vi"("type of dialog (OK msg:1)"=w244, "error in (no error)"=w243) -> ()  [unwired: 3 in, 5 out]
            }
          }
        }
        frame "Wavefront sensor" {
          n120 = stacked-sequence {
            frame #0 {
              w252 = T8 3 items=["no dialog", "OK message", "continue or stop message", "OK message + warnings", "continue/stop + warnings"] ("type of dialog (OK msg:1)")
              n121 = local write "Camera image"(u32[][] [] ("Camera image")) -> ()
              n122 = call-poly <vilib>:"DAQmx Create Virtual Channel.vi"("physical channels"=tag "Dev1/ao5") -> ("task out"=w256:refnum<k21>, "error out"=w257:errorcluster)  [unwired: 13 in]
              n123 = call-poly <vilib>:"DAQmx Write.vi"("task/channels in"=w256, "auto start"=TRUE, "data"=1.0 ("AO 5"), "error in"=w257) -> ("task out"=w254:refnum<k21>, "error out"=w255:errorcluster)  [unwired: 9 in, 1 out]
              n124 = call <vilib>:"DAQmx Clear Task.vi"("task in"=w254, "error in"=w255) -> ("error out"=w253:errorcluster)  [unwired: 13 in]
              n125 = call <vilib>:"Simple Error Handler.vi"("type of dialog (OK msg:1)"=w252, "error in (no error)"=w253) -> ()  [unwired: 3 in, 5 out]
              "before correction" <- dbl[][] [] ("before correction")
              "after correction" <- dbl[][] [] ("after correction")
            }
            frame #1 {
              n126 = case shown="True" "Boolean 2" {
                frame False {
                  n127 = stacked-sequence {
                    seq-local: [w264 _ _] -> [_ w342 _]
                    seq-local: [w263 _ _] -> [_ w341 _]
                    frame #0 {
                      w273 = -90.0  # Em Fast Galvo Phase
                      w323 = 1.0  # Em Slow Galvo (Hz)
                      w321 = 1.0  # Ex Slow Galvo (Hz)
                      w269 = 0.1175  # Amplitude (V)
                      w320 = 500.0  # Ex Fast Galvo (Hz)
                      w271 = 0.14  # Amplitude (V)
                      w319 = 500.0  # Pockels Cell Frequency (Hz)
                      w317 = 500.0  # Em Fast Galvo (Hz)
                      w272 = 90.0  # Em Slow Galvo Phase
                      w313 = 90.0  # Ex Slow Galvo Phase
                      w314 = 90.0  # Ex Fast Galvo Phase
                      w310 = 10280 items=["Rising"=10280, "Falling"=10171] ("edge")
                      w305 = 10178 items=["Finite Samples"=10178, "Continuous Samples"=10123, "Hardware Timed Single Point"=12522] ("sample mode")
                      n128 = Bundle By Name(cluster=T2 {"Galvo/Pockels Cell Sampling Info"=1000000.0, "#s"=500000.0} ("Sampling Info"), "#s"="Exp Time") -> (w261:T2)
                      n129 = Multiply(x="Scale factor", y=w269) -> (x*y=w268:dbl)
                      n130 = Multiply(x=w271, y="Scale factor") -> (x*y=w267:dbl)
                      n131 = Multiply(x="Power%(0-100)", y=0.0137 ("data")) -> (x*y=w318:dbl)
                      n132 = expression code="(x/180.0)*pi" "degrees to radians"(0.0 ("Ex Theta")) -> (w277:dbl)
                      n133 = expression code="(x/180.0)*pi" "degrees to radians"(0.3 ("Em Theta")) -> (w274:dbl)
                      n134 = call <vilib>:"Sine Waveform.vi"("sampling info"=w261, "reset signal"=TRUE, "phase"=w314, "amplitude"=w267, "frequency"=w320) -> ("signal out"=w289:waveform(dbl))  [unwired: 5 in, 1 out]
                      n135 = call <vilib>:"Triangle Waveform.vi"("sampling info"=w261, "reset signal"=TRUE, "phase"=w313, "amplitude"=w268, "frequency"=w321) -> ("signal out"=w290:waveform(dbl))  [unwired: 5 in, 1 out]
                      n136 = call <vilib>:"Triangle Waveform.vi"("sampling info"=w261, "reset signal"=TRUE, "phase"=w272, "amplitude"=w268, "frequency"=w323) -> ("signal out"=w281:waveform(dbl))  [unwired: 5 in, 1 out]
                      n137 = call <vilib>:"Sine Waveform.vi"("sampling info"=w261, "reset signal"=TRUE, "phase"=w273, "amplitude"=w267, "frequency"=w317) -> ("signal out"=w276:waveform(dbl))  [unwired: 5 in, 1 out]
                      n138 = Square(x=w318) -> (x^2=w292:dbl)
                      n139 = call-poly <vilib>:"DAQmx Create Virtual Channel.vi"("physical channels"=tag "Dev1/ao0:4") -> ("task out"=w307:refnum<k21>, "error out"=w300:errorcluster)  [unwired: 13 in]
                      n140 = call-poly <vilib>:"2D Cartesian Coordinate Rotation.vi"("theta"=w277, "Y"=w290, "X"=w289) -> ("Y Out"=w286:dbl[], "X Out"=w288:dbl[])  [unwired: 6 in, 1 out]
                      n141 = call-poly <vilib>:"2D Cartesian Coordinate Rotation.vi"("theta"=w274, "Y"=w281, "X"=w276) -> ("Y Out"=w282:dbl[], "X Out"=w283:dbl[])  [unwired: 6 in, 1 out]
                      n142 = Square(x=w292) -> (x^2=w291:dbl)
                      n143 = call-poly <vilib>:"DAQmx Timing.vi"("task/channels in"=w307, "sample mode"=w305, "waveform"=w276, "error in"=w300) -> ("task out"=w301:refnum<k21>, "error out"=w302:errorcluster)  [unwired: 10 in]
                      n144 = Bundle By Name "Build Waveform"("Y"=w288) -> (w287:waveform(dbl))  [unwired: 1 in]
                      n145 = Bundle By Name "Build Waveform"("Y"=w286) -> (w285:waveform(dbl))  [unwired: 1 in]
                      n146 = Bundle By Name "Build Waveform"("Y"=w283) -> (w279:waveform(dbl))  [unwired: 1 in]
                      n147 = Bundle By Name "Build Waveform"("Y"=w282) -> (w280:waveform(dbl))  [unwired: 1 in]
                      n148 = call <vilib>:"Sine Waveform.vi"("sampling info"=w261, "reset signal"=TRUE, "phase"=135.0, "amplitude"=w291, "frequency"=w319) -> ("signal out"=w316:waveform(dbl))  [unwired: 5 in, 1 out]
                      n149 = Absolute Value(x=w316) -> (abs(x)=w294:waveform(dbl))
                      n150 = Square Root(x=w294) -> (sqrt(x)=w293:waveform(dbl))
                      n151 = Square Root(x=w293) -> (sqrt(x)=w284:waveform(dbl))
                      n152 = Build Array "Build Array"(w287, w285, w279, w280, w284) -> (w308:waveform(dbl)[])
                      n153 = call-poly <vilib>:"DAQmx Write.vi"("task/channels in"=w301, "auto start"=FALSE, "data"=w308, "error in"=w302) -> ("task out"=w303:refnum<k21>, "error out"=w304:errorcluster)  [unwired: 9 in, 1 out]
                      n154 = call-poly <vilib>:"DAQmx Trigger.vi"("task/channels in"=w303, "source"=tag "/Dev1/PFI1", "edge"=w310, "error in"=w304) -> ("task out"=w311:refnum<k21>, "error out"=w312:errorcluster)  [unwired: 10 in]
                      n155 = call <vilib>:"DAQmx Start Task.vi"("task/channels in"=w311, "error in"=w312) -> ("task out"=w264:refnum<k21>, "error out"=w263:errorcluster)  [unwired: 12 in]
                    }
                    frame #1 {
                      n156 = flat-sequence {
                        tunnel: [w352] -> w333
                        tunnel: [w351] -> w331
                        tunnel: [w350] -> w329
                        tunnel: [w349] -> w327
                        tunnel: [w345] -> w325
                        tunnel: [w344] -> w324
                        tunnel: w333 -> [w377]
                        tunnel: [w377] -> w332
                        tunnel: w331 -> [w376]
                        tunnel: [w376] -> w330
                        tunnel: w329 -> [w375]
                        tunnel: [w375] -> w328
                        tunnel: w327 -> [w374]
                        tunnel: [w374] -> w326
                        tunnel: w325 -> [w367]
                        tunnel: w324 -> [w366]
                        tunnel: w342 -> [w388]
                        tunnel: w341 -> [w387]
                        tunnel: [w381] -> w340
                        tunnel: [w386] -> w339
                        tunnel: w332 -> [w386]
                        tunnel: [w385] -> w338
                        tunnel: w330 -> [w385]
                        tunnel: w328 -> [w378]
                        tunnel: w326 -> [w379]
                        tunnel: [w383] -> w334
                        tunnel: w340 -> [w404]
                        tunnel: w339 -> [w418]
                        tunnel: w338 -> [w420]
                        tunnel: [w406] -> w337
                        tunnel: [w401] -> w336
                        tunnel: [w405] -> w335
                        tunnel: w334 -> [w403]
                        tunnel: w337 -> [w430]
                        tunnel: w336 -> [w428]
                        tunnel: w335 -> [w426]
                        frame #0 {
                          n157 = call <vilib>:"Haso ctor serial number.vi"("Serial number"="Haso serial number") -> ("error out"=w363:errorcluster, "Haso"=w364:T9)  [unwired: 5 in]
                          n158 = local read "Exp Time"() -> (w343:u32)
                          n159 = call "Haso camera.vi"("error in (no error)"=w363, "Haso"=w364) -> ("error out"=w354:errorcluster, "camera"=w362:T10, "Haso (dup)"=w355:T9)  [unwired: 3 in]
                          n160 = call <vilib>:"DataHaso ctor Haso.vi"("error in (no error)"=w354, "Haso"=w355) -> ("error out"=w353:errorcluster, "Haso (dup)"=w351:T9, "Data Haso"=w352:T5)  [unwired: 3 in]
                          n161 = call <vilib>:"Camera Get Preferences.vi"("error in (no error)"=w353, "Camera"=w362) -> ("error out"=w361:errorcluster, "Camera Preferences"=w359:T11, "Camera (dup)"=w360:T10)  [unwired: 3 in]
                          n162 = Bundle By Name(cluster=w359, "Exposure duration specified (µs)"=w343, "Timeout delay (ms)"=u32 2000, "Trigger type"=enum16{"Internal", "TTL", "Software"}."Internal") -> (w358:T11)
                          n163 = call "Camera Set Preferences.vi"("error in (no error)"=w361, "Camera Preferences"=w358, "Camera"=w360) -> ("error out"=w356:errorcluster, "Camera (dup)"=w357:T10)  [unwired: 3 in]
                          n164 = call-poly <vilib>:"DAQmx Create Virtual Channel.vi"("lines"=tag "Dev1/port0/line2") -> ("task out"=w344:refnum<k21>, "error out"=w345:errorcluster)  [unwired: 13 in]
                          n165 = call <vilib>:"Camera Start.vi"("error in (no error)"=w356, "camera"=w357) -> ("error out"=w349:errorcluster, "camera (dup)"=w350:T10)  [unwired: 4 in]
                        }
                        frame #1 {
                          w370 = T8 3 items=["no dialog", "OK message", "continue or stop message", "OK message + warnings", "continue/stop + warnings"] ("type of dialog (OK msg:1)")
                          n166 = call-poly <vilib>:"DAQmx Write.vi"("task/channels in"=w366, "auto start"=TRUE, "data"=TRUE ("Shutter"), "error in"=w367) -> ("task out"=w369:refnum<k21>, "error out"=w368:errorcluster)  [unwired: 9 in, 1 out]
                          n167 = call <vilib>:"DAQmx Clear Task.vi"("task in"=w369, "error in"=w368) -> ("error out"=w373:errorcluster)  [unwired: 13 in]
                          n168 = call <vilib>:"Simple Error Handler.vi"("type of dialog (OK msg:1)"=w370, "error in (no error)"=w373) -> ()  [unwired: 3 in, 5 out]
                        }
                        frame #2 {
                          w389 = T8 3 items=["no dialog", "OK message", "continue or stop message", "OK message + warnings", "continue/stop + warnings"] ("type of dialog (OK msg:1)")
                          n169 = while {
                            tunnel: w388 -> [w397]
                            tunnel: [w395] -> w391
                            tunnel: w387 -> [w396]
                            tunnel: [w394] -> w392
                            stop <- w393 stop-if-true
                            n170 = call <vilib>:"DAQmx Is Task Done.vi"("task/channels in"=w397, "error in"=w396) -> ("task out"=w395:refnum<k21>, "task done?"=w393:bool, "error out"=w394:errorcluster)  [unwired: 11 in]
                          }
                          n171 = call <vilib>:"Camera Get image.vi"("error in (no error)"=w379, "camera"=w378) -> ("error out"=w382:errorcluster, "Image"=w384:T12)  [unwired: 3 in, 1 out]
                          n172 = call "Image get data.vi"("error in (no error)"=w382, "Image Compat"=w384) -> ("error out"=w381:errorcluster, "Array"=→"Camera image":u32[][], "Image Compat (dup)"=w383:T12)  [unwired: 3 in]
                          n173 = call <vilib>:"DAQmx Clear Task.vi"("task in"=w391, "error in"=w392) -> ("error out"=w390:errorcluster)  [unwired: 13 in]
                          n174 = call <vilib>:"Simple Error Handler.vi"("type of dialog (OK msg:1)"=w389, "error in (no error)"=w390) -> ()  [unwired: 3 in, 5 out]
                        }
                        frame #3 {
                          n175 = call <vilib>:"Haso compute slopes.vi"("error in (no error)"=w404, "Image Compat"=w403, "Haso"=w420) -> ("error out"=w417:errorcluster, "Data Haso"=w419:T5, "Haso (dup)"=w405:T9)  [unwired: 1 in, 1 out]
                          n176 = call <vilib>:"DataHaso Equal.vi"("error in (no error)"=w417, "Data Haso 2"=w419, "Data Haso 1"=w418) -> ("error out"=w413:errorcluster, "Data Haso 1 (dup)"=w416:T5)  [unwired: 2 in, 1 out]
                          n177 = call <vilib>:"DataHaso parameters.vi"("error in (no error)"=w413, "Data Haso"=w416) -> ("error out"=w412:errorcluster, "Parameters"=→"Parameters":T1, "Data Haso (dup)"=w414:T5)  [unwired: 3 in]
                          n178 = Bundle(cluster=T3 {"Filtre tilt X"=FALSE, "Filtre tilt Y"=FALSE, "Filtre courbure"=FALSE} ("Filtre"), "Filtre tilt X"="Filter x tilt", "Filtre tilt Y"="Filter y tilt", "Filtre courbure"="Curvature filter") -> (w421:T3)
                          n179 = control-ref of="before correction"() -> (w408:refnum<vi>)
                          n180 = call "DataHaso filter tilt or curvature.vi"("error in (no error)"=w412, "Filter (default: all true)"=w421, "Data Haso"=w414) -> ("error out"=w410:errorcluster, "Data Haso (dup)"=w411:T5)  [unwired: 3 in]
                          n181 = call "DataHaso phase.vi"("error in (no error)"=w410, "Data Haso"=w411) -> ("error out"=w407:errorcluster, "Phase (µm)"=w409:i32, "Data Haso (dup)"=w406:T5)  [unwired: 3 in]
                          n182 = call "Formatter Intensity Graph.vi"("error in (no error)"=w407, "Intensity Graph"=w408, "Surface with pupil"=w409) -> ("error out"=w402:errorcluster, "Surface with pupil (dup)"=w400:i32)  [unwired: 2 in, 1 out]
                          n183 = call <vilib>:"Surface with pupil get stats.vi"("error in (no error)"=w402, "Surface Avec Pupille"=w400) -> ("error out"=w401:errorcluster, "PV"=→"PV":sgl, "RMS"=→"RMS":dbl)  [unwired: 2 in, 1 out]
                        }
                        frame #4 {
                          n184 = call <vilib>:"Haso dtor.vi"("haso"=w426) -> ("error out"=w427:errorcluster)  [unwired: 6 in]
                          n185 = call "DataHaso dtor.vi"("Data Haso"=w430) -> ("error out"=w429:errorcluster)  [unwired: 6 in]
                          n186 = Merge Errors(w427, w429, w428) -> (w431:errorcluster)
                          n187 = call <vilib>:"Simple Error Handler.vi"("error in (no error)"=w431) -> ()  [unwired: 4 in, 5 out]
                        }
                      }
                    }
                    frame #2 {
                      w433 = T8 3 items=["no dialog", "OK message", "continue or stop message", "OK message + warnings", "continue/stop + warnings"] ("type of dialog (OK msg:1)")
                      w442 = T8 3 items=["no dialog", "OK message", "continue or stop message", "OK message + warnings", "continue/stop + warnings"] ("type of dialog (OK msg:1)")
                      n188 = call-poly <vilib>:"DAQmx Create Virtual Channel.vi"("lines"=tag "Dev1/port0/line2") -> ("task out"=w446:refnum<k21>, "error out"=w445:errorcluster)  [unwired: 13 in]
                      n189 = call-poly <vilib>:"DAQmx Create Virtual Channel.vi"("lines"=tag "Dev1/port0/line1") -> ("task out"=w437:refnum<k21>, "error out"=w436:errorcluster)  [unwired: 13 in]
                      n190 = call-poly <vilib>:"DAQmx Write.vi"("task/channels in"=w446, "auto start"=TRUE, "data"=FALSE ("Shutter"), "error in"=w445) -> ("task out"=w448:refnum<k21>, "error out"=w449:errorcluster)  [unwired: 9 in, 1 out]
                      n191 = call-poly <vilib>:"DAQmx Write.vi"("task/channels in"=w437, "auto start"=TRUE, "data"=FALSE ("Shutter"), "error in"=w436) -> ("task out"=w439:refnum<k21>, "error out"=w440:errorcluster)  [unwired: 9 in, 1 out]
                      n192 = call <vilib>:"DAQmx Clear Task.vi"("task in"=w448, "error in"=w449) -> ("error out"=w443:errorcluster)  [unwired: 13 in]
                      n193 = call <vilib>:"DAQmx Clear Task.vi"("task in"=w439, "error in"=w440) -> ("error out"=w434:errorcluster)  [unwired: 13 in]
                      n194 = call <vilib>:"Simple Error Handler.vi"("type of dialog (OK msg:1)"=w442, "error in (no error)"=w443) -> ()  [unwired: 3 in, 5 out]
                      n195 = call <vilib>:"Simple Error Handler.vi"("type of dialog (OK msg:1)"=w433, "error in (no error)"=w434) -> ()  [unwired: 3 in, 5 out]
                    }
                  }
                }
                frame True {
                  n196 = stacked-sequence {
                    seq-local: [_ w538 _ _ _] -> [_ _ _ w747 _]
                    seq-local: [_ w537 _ _ _] -> [_ _ _ w746 _]
                    seq-local: [_ w534 _ _ _] -> [_ _ _ w738 _]
                    seq-local: [_ w535 _ _ _] -> [_ _ _ w750 _]
                    seq-local: [_ w536 _ _ _] -> [_ _ _ w751 _]
                    seq-local: [w454 _ _ _ _] -> [_ w520 _ _ _]
                    seq-local: [w453 _ _ _ _] -> [_ w521 _ _ _]
                    seq-local: [_ _ w678 _ _] -> [_ _ _ w749 _]
                    seq-local: [_ _ w677 _ _] -> [_ _ _ w748 _]
                    seq-local: [_ w514 _ _ _] -> [_ _ _ w739 _]
                    frame #0 {
                      w463 = -90.0  # Em Fast Galvo Phase
                      w513 = 1.0  # Em Slow Galvo (Hz)
                      w511 = 1.0  # Ex Slow Galvo (Hz)
                      w460 = 0.1175  # Amplitude (V)
                      w510 = 500.0  # Ex Fast Galvo (Hz)
                      w461 = 0.14  # Amplitude (V)
                      w509 = 500.0  # Pockels Cell Frequency (Hz)
                      w507 = 500.0  # Em Fast Galvo (Hz)
                      w462 = 90.0  # Em Slow Galvo Phase
                      w503 = 90.0  # Ex Slow Galvo Phase
                      w504 = 90.0  # Ex Fast Galvo Phase
                      w500 = 10280 items=["Rising"=10280, "Falling"=10171] ("edge")
                      w495 = 10178 items=["Finite Samples"=10178, "Continuous Samples"=10123, "Hardware Timed Single Point"=12522] ("sample mode")
                      n197 = local read "Exp Time"() -> (w450:u32)
                      n198 = Bundle By Name(cluster=T2 {"Galvo/Pockels Cell Sampling Info"=1000000.0, "#s"=500000.0} ("Sampling Info"), "#s"=w450) -> (w451:T2)
                      n199 = local read "Scale factor"() -> (w455:u16)
                      n200 = local read "Power%(0-100)"() -> (w456:dbl)
                      n201 = Multiply(x=w455, y=w460) -> (x*y=w459:dbl)
                      n202 = Multiply(x=w461, y=w455) -> (x*y=w458:dbl)
                      n203 = expression code="(x/180.0)*pi" "degrees to radians"(0.0 ("Ex Theta")) -> (w467:dbl)
                      n204 = expression code="(x/180.0)*pi" "degrees to radians"(0.3 ("Em Theta")) -> (w464:dbl)
                      n205 = call <vilib>:"Sine Waveform.vi"("sampling info"=w451, "reset signal"=TRUE, "phase"=w504, "amplitude"=w458, "frequency"=w510) -> ("signal out"=w479:waveform(dbl))  [unwired: 5 in, 1 out]
                      n206 = call <vilib>:"Triangle Waveform.vi"("sampling info"=w451, "reset signal"=TRUE, "phase"=w503, "amplitude"=w459, "frequency"=w511) -> ("signal out"=w480:waveform(dbl))  [unwired: 5 in, 1 out]
                      n207 = call <vilib>:"Triangle Waveform.vi"("sampling info"=w451, "reset signal"=TRUE, "phase"=w462, "amplitude"=w459, "frequency"=w513) -> ("signal out"=w471:waveform(dbl))  [unwired: 5 in, 1 out]
                      n208 = Multiply(x=w456, y=0.0137 ("data")) -> (x*y=w508:dbl)
                      n209 = call <vilib>:"Sine Waveform.vi"("sampling info"=w451, "reset signal"=TRUE, "phase"=w463, "amplitude"=w458, "frequency"=w507) -> ("signal out"=w466:waveform(dbl))  [unwired: 5 in, 1 out]
                      n210 = call-poly <vilib>:"DAQmx Create Virtual Channel.vi"("physical channels"=tag "Dev1/ao0:4") -> ("task out"=w497:refnum<k21>, "error out"=w490:errorcluster)  [unwired: 13 in]
                      n211 = call-poly <vilib>:"2D Cartesian Coordinate Rotation.vi"("theta"=w467, "Y"=w480, "X"=w479) -> ("Y Out"=w476:dbl[], "X Out"=w478:dbl[])  [unwired: 6 in, 1 out]
                      n212 = call-poly <vilib>:"2D Cartesian Coordinate Rotation.vi"("theta"=w464, "Y"=w471, "X"=w466) -> ("Y Out"=w472:dbl[], "X Out"=w473:dbl[])  [unwired: 6 in, 1 out]
                      n213 = Square(x=w508) -> (x^2=w482:dbl)
                      n214 = call-poly <vilib>:"DAQmx Timing.vi"("task/channels in"=w497, "sample mode"=w495, "waveform"=w466, "error in"=w490) -> ("task out"=w491:refnum<k21>, "error out"=w492:errorcluster)  [unwired: 10 in]
                      n215 = Bundle By Name "Build Waveform"("Y"=w478) -> (w477:waveform(dbl))  [unwired: 1 in]
                      n216 = Bundle By Name "Build Waveform"("Y"=w476) -> (w475:waveform(dbl))  [unwired: 1 in]
                      n217 = Bundle By Name "Build Waveform"("Y"=w473) -> (w469:waveform(dbl))  [unwired: 1 in]
                      n218 = Bundle By Name "Build Waveform"("Y"=w472) -> (w470:waveform(dbl))  [unwired: 1 in]
                      n219 = Square(x=w482) -> (x^2=w481:dbl)
                      n220 = call <vilib>:"Sine Waveform.vi"("sampling info"=w451, "reset signal"=TRUE, "phase"=135.0, "amplitude"=w481, "frequency"=w509) -> ("signal out"=w506:waveform(dbl))  [unwired: 5 in, 1 out]
                      n221 = Absolute Value(x=w506) -> (abs(x)=w484:waveform(dbl))
                      n222 = Square Root(x=w484) -> (sqrt(x)=w483:waveform(dbl))
                      n223 = Square Root(x=w483) -> (sqrt(x)=w474:waveform(dbl))
                      n224 = Build Array "Build Array"(w477, w475, w469, w470, w474) -> (w498:waveform(dbl)[])
                      n225 = call-poly <vilib>:"DAQmx Write.vi"("task/channels in"=w491, "auto start"=FALSE, "data"=w498, "error in"=w492) -> ("task out"=w493:refnum<k21>, "error out"=w494:errorcluster)  [unwired: 9 in, 1 out]
                      n226 = call-poly <vilib>:"DAQmx Trigger.vi"("task/channels in"=w493, "source"=tag "/Dev1/PFI1", "edge"=w500, "error in"=w494) -> ("task out"=w501:refnum<k21>, "error out"=w502:errorcluster)  [unwired: 10 in]
                      n227 = call <vilib>:"DAQmx Start Task.vi"("task/channels in"=w501, "error in"=w502) -> ("task out"=w454:refnum<k21>, "error out"=w453:errorcluster)  [unwired: 12 in]
                    }
                    frame #1 {
                      # "camera"
                      # "haso"
                      # "dhaso"
                      # "casao"
                      # "dhaso"
                      n228 = flat-sequence {
                        tunnel: [w548] -> w529
                        tunnel: [w560] -> w527
                        tunnel: [w559] -> w525
                        tunnel: [w557] -> w522
                        tunnel: [w546] -> w517
                        tunnel: w529 -> [w592]
                        tunnel: [w592] -> w528
                        tunnel: w527 -> [w591]
                        tunnel: [w591] -> w526
                        tunnel: w525 -> [w590]
                        tunnel: [w590] -> w524
                        tunnel: [w580] -> w523
                        tunnel: w522 -> [w580]
                        tunnel: [w579] -> w518
                        tunnel: w517 -> [w579]
                        tunnel: [w597] -> w543
                        tunnel: w528 -> [w605]
                        tunnel: [w614] -> w542
                        tunnel: w526 -> [w614]
                        tunnel: [w613] -> w541
                        tunnel: w524 -> [w613]
                        tunnel: [w598] -> w540
                        tunnel: [w599] -> w539
                        tunnel: w523 -> [w600]
                        tunnel: w521 -> [w608]
                        tunnel: w520 -> [w607]
                        tunnel: w518 -> [w606]
                        tunnel: [w595] -> w516
                        tunnel: w543 -> [w648]
                        tunnel: w542 -> [w644]
                        tunnel: w541 -> [w647]
                        tunnel: w540 -> [w646]
                        tunnel: w539 -> [w625]
                        tunnel: [w641] -> w533
                        tunnel: [w640] -> w532
                        tunnel: [w639] -> w531
                        tunnel: [w626] -> w530
                        tunnel: [w625] -> w519
                        tunnel: w516 -> [w624]
                        tunnel: [w624] -> w515
                        tunnel: [w660] -> w537
                        tunnel: [w670] -> w534
                        tunnel: [w671] -> w538
                        tunnel: [w672] -> w535
                        tunnel: [w673] -> w536
                        tunnel: w533 -> [w673]
                        tunnel: w532 -> [w672]
                        tunnel: w531 -> [w671]
                        tunnel: w530 -> [w670]
                        tunnel: w519 -> [w660]
                        tunnel: [w659] -> w514
                        tunnel: w515 -> [w659]
                        frame #0 {
                          n229 = local read "Haso serial number"() -> (w563:u32)
                          n230 = call "Casao ctor.vi"("Init mirrror hardware (default true)"=TRUE, "Mirror config file path"="Phase modulator config file path", "Haso serial number"=w563) -> ("error out"=w577:errorcluster, "Casao"=w578:T14)  [unwired: 5 in]
                          n231 = call "Casao get CasaoMatrix.vi"("error in (no error)"=w577, "Casao"=w578) -> ("error out"=w576:errorcluster, "Casao matrix"=w574:T15, "Casao (dup)"=w571:T14)  [unwired: 3 in]
                          n232 = call "CasaoMatrix Load interaction matrix.vi"("error in (no error)"=w576, "Path"="Matrix path", "Casao matrix"=w574) -> ("error out"=w575:errorcluster, "Casao matrix (dup)"=w573:T15)  [unwired: 1 in, 2 out]
                          n233 = call "CasaoMatrix Compute MC.vi"("error in (no error)"=w575, "Casao Matrix"=w573) -> ("error out"=w572:errorcluster)  [unwired: 4 in, 1 out]
                          n234 = call "Casao get PhaseModulator.vi"("error in (no error)"=w572, "Casao"=w571) -> ("error out"=w569:errorcluster, "Mirrror"=w570:T16, "Casao (dup)"=w568:T14)  [unwired: 3 in]
                          n235 = call "PhaseModul get preferences.vi"("error in (no error)"=w569, "Mirror"=w570) -> ("error out"=w561:errorcluster, "Mirror (dup)"=w560:T16)  [unwired: 3 in, 1 out]
                          n236 = call "Casao get Haso.vi"("error in (no error)"=w561, "Casao"=w568) -> ("error out"=w565:errorcluster, "Haso"=w567:T9, "Casao (dup)"=w566:T14)  [unwired: 3 in]
                          n237 = call "Haso camera.vi"("error in (no error)"=w565, "Haso"=w567) -> ("error out"=w556:errorcluster, "camera"=w554:T10, "Haso (dup)"=w557:T9)  [unwired: 3 in]
                          n238 = call "Casao Set Preferences.vi"("error in (no error)"=w565, "Loop preferences"=T4 {"Filter tilt on measurement (closed loop)"=FALSE, "Correction gain (closed loop)"=0.5, "Limit of subapertures off in CGP (%)"=0.0, "Limit of saturated actuators (%)"=0.0}, "Casao"=w566) -> ("Casao (dup)"=w559:T14)  [unwired: 3 in, 1 out]
                          n239 = call <vilib>:"Camera Get Preferences.vi"("error in (no error)"=w556, "Camera"=w554) -> ("error out"=w555:errorcluster, "Camera Preferences"=w552:T11, "Camera (dup)"=w553:T10)  [unwired: 3 in]
                          n240 = local read "Exp Time"() -> (w544:u32)
                          n241 = Bundle By Name(cluster=w552, "Exposure duration specified (µs)"=w544, "Trigger type"=enum16{"Internal", "TTL", "Software"}."Internal") -> (w551:T11)
                          n242 = call "Camera Set Preferences.vi"("error in (no error)"=w555, "Camera Preferences"=w551, "Camera"=w553) -> ("error out"=w549:errorcluster, "Camera (dup)"=w547:T10)  [unwired: 3 in]
                          n243 = call <vilib>:"Camera Start.vi"("error in (no error)"=w549, "camera"=w547) -> ("error out"=w548:errorcluster, "camera (dup)"=w546:T10)  [unwired: 4 in]
                        }
                        frame #1 {
                          w588 = T8 3 items=["no dialog", "OK message", "continue or stop message", "OK message + warnings", "continue/stop + warnings"] ("type of dialog (OK msg:1)")
                          # "casao"
                          # "mirror"
                          # "haso"
                          n244 = call-poly <vilib>:"DAQmx Create Virtual Channel.vi"("lines"=tag "Dev1/port0/line2") -> ("task out"=w584:refnum<k21>, "error out"=w585:errorcluster)  [unwired: 13 in]
                          n245 = call-poly <vilib>:"DAQmx Write.vi"("task/channels in"=w584, "auto start"=TRUE, "data"=TRUE ("Shutter"), "error in"=w585) -> ("task out"=w582:refnum<k21>, "error out"=w581:errorcluster)  [unwired: 9 in, 1 out]
                          n246 = call <vilib>:"DAQmx Clear Task.vi"("task in"=w582, "error in"=w581) -> ("error out"=w587:errorcluster)  [unwired: 13 in]
                          n247 = call <vilib>:"Simple Error Handler.vi"("type of dialog (OK msg:1)"=w588, "error in (no error)"=w587) -> ()  [unwired: 3 in, 5 out]
                        }
                        frame #2 {
                          w609 = T8 3 items=["no dialog", "OK message", "continue or stop message", "OK message + warnings", "continue/stop + warnings"] ("type of dialog (OK msg:1)")
                          # "dhaso"
                          n248 = call <vilib>:"Camera Get image.vi"("error in (no error)"=w605, "camera"=w606) -> ("error out"=w594:errorcluster, "Image"=w604:T12, "camera (dup)"=w596:T10)  [unwired: 3 in]
                          n249 = call <vilib>:"Camera Stop.vi"("error in (no error)"=w594, "camera"=w596) -> ("error out"=w593:errorcluster, "camera (dup)"=w595:T10)  [unwired: 4 in]
                          n250 = call "Image get data.vi"("error in (no error)"=w593, "Image Compat"=w604) -> ("error out"=w601:errorcluster, "Array"=w603:u32[][], "Image Compat (dup)"=w602:T12)  [unwired: 3 in]
                          n251 = local write "Camera image"(w603) -> ()
                          n252 = call <vilib>:"Haso compute slopes.vi"("error in (no error)"=w601, "Image Compat"=w602, "Haso"=w600) -> ("error out"=w597:errorcluster, "Data Haso"=w598:T5, "Haso (dup)"=w599:T9)  [unwired: 1 in, 1 out]
                          n253 = while {
                            tunnel: [w619] -> w611
                            tunnel: [w618] -> w612
                            tunnel: w608 -> [w616]
                            tunnel: w607 -> [w615]
                            stop <- w617 stop-if-true
                            n254 = call <vilib>:"DAQmx Is Task Done.vi"("task/channels in"=w615, "error in"=w616) -> ("task out"=w619:refnum<k21>, "task done?"=w617:bool, "error out"=w618:errorcluster)  [unwired: 11 in]
                          }
                          n255 = call <vilib>:"DAQmx Clear Task.vi"("task in"=w611, "error in"=w612) -> ("error out"=w610:errorcluster)  [unwired: 13 in]
                          n256 = call <vilib>:"Simple Error Handler.vi"("type of dialog (OK msg:1)"=w609, "error in (no error)"=w610) -> ()  [unwired: 3 in, 5 out]
                        }
                        frame #3 {
                          # "haso"
                          # "dhaso"
                          # "casao"
                          n257 = call "DataHaso ctor copie.vi"("error in (no error)"=w648, "DataHaso"=w646) -> ("error out"=w637:errorcluster, "new DataHaso"=w638:T5)  [unwired: 3 in, 1 out]
                          n258 = local read "Curvature filter"() -> (w630:bool)
                          n259 = call <vilib>:"DataHaso parameters.vi"("error in (no error)"=w637, "Data Haso"=w638) -> ("error out"=w634:errorcluster, "Parameters"=w636:T1, "Data Haso (dup)"=w635:T5)  [unwired: 3 in]
                          n260 = local read "Filter x tilt"() -> (w632:bool)
                          n261 = local read "Filter y tilt"() -> (w631:bool)
                          n262 = local write "Parameters"(w636) -> ()
                          n263 = Bundle By Name(cluster=T3 {"Filtre tilt X"=FALSE, "Filtre tilt Y"=FALSE, "Filtre courbure"=FALSE} ("Filtre"), "Filtre tilt X"=w632, "Filtre tilt Y"=w631, "Filtre courbure"=w630) -> (w629:T3)
                          n264 = Bundle By Name(cluster=T7 {"Target for tilt"=0, "Target for focus"=0, "Target for all other aberrations"=0} ("References"), "Target for tilt"=w646, "Target for focus"=w646) -> (w656:T7)
                          n265 = call "DataHaso filter tilt or curvature.vi"("error in (no error)"=w634, "Filter (default: all true)"=w629, "Data Haso"=w635) -> ("error out"=w628:errorcluster, "Data Haso (dup)"=w627:T5)  [unwired: 3 in]
                          n266 = call "DataHaso ctor copie.vi"("error in (no error)"=w648, "DataHaso"=w646) -> ("error out"=w655:errorcluster, "new DataHaso"=w657:T5)  [unwired: 3 in, 1 out]
                          n267 = control-ref of="before correction"() -> (w645:refnum<vi>)
                          n268 = call "Casao Compute target.vi"("error in (no error)"=w655, "Targets"=w656, "DataHaso"=w657, "Casao"=w647) -> ("error out"=w649:errorcluster, "DataHaso (dup)"=w641:T5, "Casao (dup)"=w650:T14)  [unwired: 1 out]
                          n269 = call "DataHaso phase.vi"("error in (no error)"=w628, "Data Haso"=w627) -> ("error out"=w653:errorcluster, "Phase (µm)"=w654:i32, "Data Haso (dup)"=w639:T5)  [unwired: 3 in]
                          n270 = call "Formatter Intensity Graph.vi"("error in (no error)"=w653, "Intensity Graph"=w645, "Surface with pupil"=w654) -> ("error out"=w623:errorcluster, "Surface with pupil (dup)"=w622:i32)  [unwired: 2 in, 1 out]
                          n271 = Bundle By Name(cluster=T6 {"Measurement"=0, "Target"=0, "Manual target"=0} ("Slopes"), "Target"=w641, "Measurement"=w639) -> (w651:T6)
                          n272 = call <vilib>:"Surface with pupil get stats.vi"("error in (no error)"=w623, "Surface Avec Pupille"=w622) -> ("PV"=w621:sgl, "RMS"=w620:dbl)  [unwired: 2 in, 2 out]
                          n273 = local write "PV"(w621) -> ()
                          n274 = local write "RMS"(w620) -> ()
                          n275 = call "Casao get correction commands.vi"("Casao"=w650, "Slopes"=w651, "error in (no error)"=w649) -> ("Casao (dup)"=w640:T14, "Commands"=w643:sgl[], "error out"=w642:errorcluster)  [unwired: 2 in, 2 out]
                          n276 = call "PhaseModul apply command.vi"("error in (no error)"=w642, "Commands in"=w643, "Mirror"=w644) -> ("error out"=w626:errorcluster)  [unwired: 2 in, 2 out]
                        }
                        frame #4 {
                          w662 = T8 3 items=["no dialog", "OK message", "continue or stop message", "OK message + warnings", "continue/stop + warnings"] ("type of dialog (OK msg:1)")
                          # "haso"
                          # "casao"
                          n277 = call-poly <vilib>:"DAQmx Create Virtual Channel.vi"("lines"=tag "Dev1/port0/line2") -> ("task out"=w666:refnum<k21>, "error out"=w665:errorcluster)  [unwired: 13 in]
                          n278 = call-poly <vilib>:"DAQmx Write.vi"("task/channels in"=w666, "auto start"=TRUE, "data"=FALSE ("Shutter"), "error in"=w665) -> ("task out"=w668:refnum<k21>, "error out"=w669:errorcluster)  [unwired: 9 in, 1 out]
                          n279 = call <vilib>:"DAQmx Clear Task.vi"("task in"=w668, "error in"=w669) -> ("error out"=w663:errorcluster)  [unwired: 13 in]
                          n280 = call <vilib>:"Simple Error Handler.vi"("type of dialog (OK msg:1)"=w662, "error in (no error)"=w663) -> ()  [unwired: 3 in, 5 out]
                        }
                      }
                    }
                    frame #2 {
                      w687 = -90.0  # Em Fast Galvo Phase
                      w737 = 1.0  # Em Slow Galvo (Hz)
                      w735 = 1.0  # Ex Slow Galvo (Hz)
                      w684 = 0.1175  # Amplitude (V)
                      w734 = 500.0  # Ex Fast Galvo (Hz)
                      w685 = 0.14  # Amplitude (V)
                      w733 = 500.0  # Pockels Cell Frequency (Hz)
                      w731 = 500.0  # Em Fast Galvo (Hz)
                      w686 = 90.0  # Em Slow Galvo Phase
                      w727 = 90.0  # Ex Slow Galvo Phase
                      w728 = 90.0  # Ex Fast Galvo Phase
                      w724 = 10280 items=["Rising"=10280, "Falling"=10171] ("edge")
                      w719 = 10178 items=["Finite Samples"=10178, "Continuous Samples"=10123, "Hardware Timed Single Point"=12522] ("sample mode")
                      n281 = local read "Scale factor"() -> (w679:u16)
                      n282 = local read "Power%(0-100)"() -> (w680:dbl)
                      n283 = Multiply(x=w679, y=w684) -> (x*y=w683:dbl)
                      n284 = Multiply(x=w685, y=w679) -> (x*y=w682:dbl)
                      n285 = local read "Exp Time"() -> (w674:u32)
                      n286 = Bundle By Name(cluster=T2 {"Galvo/Pockels Cell Sampling Info"=1000000.0, "#s"=500000.0} ("Sampling Info"), "#s"=w674) -> (w675:T2)
                      n287 = expression code="(x/180.0)*pi" "degrees to radians"(0.0 ("Ex Theta")) -> (w691:dbl)
                      n288 = expression code="(x/180.0)*pi" "degrees to radians"(0.3 ("Em Theta")) -> (w688:dbl)
                      n289 = call <vilib>:"Sine Waveform.vi"("sampling info"=w675, "reset signal"=TRUE, "phase"=w728, "amplitude"=w682, "frequency"=w734) -> ("signal out"=w703:waveform(dbl))  [unwired: 5 in, 1 out]
                      n290 = call <vilib>:"Triangle Waveform.vi"("sampling info"=w675, "reset signal"=TRUE, "phase"=w727, "amplitude"=w683, "frequency"=w735) -> ("signal out"=w704:waveform(dbl))  [unwired: 5 in, 1 out]
                      n291 = call <vilib>:"Triangle Waveform.vi"("sampling info"=w675, "reset signal"=TRUE, "phase"=w686, "amplitude"=w683, "frequency"=w737) -> ("signal out"=w695:waveform(dbl))  [unwired: 5 in, 1 out]
                      n292 = Multiply(x=w680, y=0.0137 ("data")) -> (x*y=w732:dbl)
                      n293 = call <vilib>:"Sine Waveform.vi"("sampling info"=w675, "reset signal"=TRUE, "phase"=w687, "amplitude"=w682, "frequency"=w731) -> ("signal out"=w690:waveform(dbl))  [unwired: 5 in, 1 out]
                      n294 = call-poly <vilib>:"DAQmx Create Virtual Channel.vi"("physical channels"=tag "Dev1/ao0:4") -> ("task out"=w721:refnum<k21>, "error out"=w714:errorcluster)  [unwired: 13 in]
                      n295 = call-poly <vilib>:"2D Cartesian Coordinate Rotation.vi"("theta"=w691, "Y"=w704, "X"=w703) -> ("Y Out"=w700:dbl[], "X Out"=w702:dbl[])  [unwired: 6 in, 1 out]
                      n296 = call-poly <vilib>:"2D Cartesian Coordinate Rotation.vi"("theta"=w688, "Y"=w695, "X"=w690) -> ("Y Out"=w696:dbl[], "X Out"=w697:dbl[])  [unwired: 6 in, 1 out]
                      n297 = Square(x=w732) -> (x^2=w706:dbl)
                      n298 = call-poly <vilib>:"DAQmx Timing.vi"("task/channels in"=w721, "sample mode"=w719, "waveform"=w690, "error in"=w714) -> ("task out"=w715:refnum<k21>, "error out"=w716:errorcluster)  [unwired: 10 in]
                      n299 = Bundle By Name "Build Waveform"("Y"=w702) -> (w701:waveform(dbl))  [unwired: 1 in]
                      n300 = Bundle By Name "Build Waveform"("Y"=w700) -> (w699:waveform(dbl))  [unwired: 1 in]
                      n301 = Bundle By Name "Build Waveform"("Y"=w697) -> (w693:waveform(dbl))  [unwired: 1 in]
                      n302 = Bundle By Name "Build Waveform"("Y"=w696) -> (w694:waveform(dbl))  [unwired: 1 in]
                      n303 = Square(x=w706) -> (x^2=w705:dbl)
                      n304 = call <vilib>:"Sine Waveform.vi"("sampling info"=w675, "reset signal"=TRUE, "phase"=135.0, "amplitude"=w705, "frequency"=w733) -> ("signal out"=w730:waveform(dbl))  [unwired: 5 in, 1 out]
                      n305 = Absolute Value(x=w730) -> (abs(x)=w708:waveform(dbl))
                      n306 = Square Root(x=w708) -> (sqrt(x)=w707:waveform(dbl))
                      n307 = Square Root(x=w707) -> (sqrt(x)=w698:waveform(dbl))
                      n308 = Build Array "Build Array"(w701, w699, w693, w694, w698) -> (w722:waveform(dbl)[])
                      n309 = call-poly <vilib>:"DAQmx Write.vi"("task/channels in"=w715, "auto start"=FALSE, "data"=w722, "error in"=w716) -> ("task out"=w717:refnum<k21>, "error out"=w718:errorcluster)  [unwired: 9 in, 1 out]
                      n310 = call-poly <vilib>:"DAQmx Trigger.vi"("task/channels in"=w717, "source"=tag "/Dev1/PFI1", "edge"=w724, "error in"=w718) -> ("task out"=w725:refnum<k21>, "error out"=w726:errorcluster)  [unwired: 10 in]
                      n311 = call <vilib>:"DAQmx Start Task.vi"("task/channels in"=w725, "error in"=w726) -> ("task out"=w678:refnum<k21>, "error out"=w677:errorcluster)  [unwired: 12 in]
                    }
                    frame #3 {
                      n312 = flat-sequence {
                        tunnel: [w762] -> w741
                        tunnel: [w761] -> w740
                        tunnel: w739 -> [w760]
                        tunnel: w738 -> [w759]
                        tunnel: w749 -> [w781]
                        tunnel: w748 -> [w780]
                        tunnel: w746 -> [w779]
                        tunnel: [w774] -> w745
                        tunnel: [w777] -> w744
                        tunnel: [w779] -> w743
                        tunnel: w741 -> [w773]
                        tunnel: w740 -> [w772]
                        tunnel: w745 -> [w802]
                        tunnel: w744 -> [w801]
                        tunnel: w743 -> [w800]
                        tunnel: [w795] -> w742
                        tunnel: w751 -> [w819]
                        tunnel: w750 -> [w818]
                        tunnel: w747 -> [w817]
                        tunnel: w742 -> [w816]
                        frame #0 {
                          w764 = T8 3 items=["no dialog", "OK message", "continue or stop message", "OK message + warnings", "continue/stop + warnings"] ("type of dialog (OK msg:1)")
                          n313 = local read "Exp Time"() -> (w752:u32)
                          n314 = call <vilib>:"Camera Get Preferences.vi"("error in (no error)"=w759, "Camera"=w760) -> ("error out"=w758:errorcluster, "Camera Preferences"=w754:T11, "Camera (dup)"=w755:T10)  [unwired: 3 in]
                          n315 = Bundle By Name(cluster=w754, "Exposure duration specified (µs)"=w752) -> (w753:T11)
                          n316 = call-poly <vilib>:"DAQmx Create Virtual Channel.vi"("lines"=tag "Dev1/port0/line2") -> ("task out"=w768:refnum<k21>, "error out"=w767:errorcluster)  [unwired: 13 in]
                          n317 = call "Camera Set Preferences.vi"("error in (no error)"=w758, "Camera Preferences"=w753, "Camera"=w755) -> ("error out"=w757:errorcluster, "Camera (dup)"=w756:T10)  [unwired: 3 in]
                          n318 = call <vilib>:"Camera Start.vi"("error in (no error)"=w757, "camera"=w756) -> ("error out"=w761:errorcluster, "camera (dup)"=w762:T10)  [unwired: 4 in]
                          n319 = call-poly <vilib>:"DAQmx Write.vi"("task/channels in"=w768, "auto start"=TRUE, "data"=TRUE ("Shutter"), "error in"=w767) -> ("task out"=w770:refnum<k21>, "error out"=w771:errorcluster)  [unwired: 9 in, 1 out]
                          n320 = call <vilib>:"DAQmx Clear Task.vi"("task in"=w770, "error in"=w771) -> ("error out"=w765:errorcluster)  [unwired: 13 in]
                          n321 = call <vilib>:"Simple Error Handler.vi"("type of dialog (OK msg:1)"=w764, "error in (no error)"=w765) -> ()  [unwired: 3 in, 5 out]
                        }
                        frame #1 {
                          w782 = T8 3 items=["no dialog", "OK message", "continue or stop message", "OK message + warnings", "continue/stop + warnings"] ("type of dialog (OK msg:1)")
                          n322 = while {
                            tunnel: w781 -> [w790]
                            tunnel: [w788] -> w784
                            tunnel: w780 -> [w789]
                            tunnel: [w787] -> w785
                            stop <- w786 stop-if-true
                            n323 = call <vilib>:"DAQmx Is Task Done.vi"("task/channels in"=w790, "error in"=w789) -> ("task out"=w788:refnum<k21>, "task done?"=w786:bool, "error out"=w787:errorcluster)  [unwired: 11 in]
                          }
                          n324 = call <vilib>:"DAQmx Clear Task.vi"("task in"=w784, "error in"=w785) -> ("error out"=w783:errorcluster)  [unwired: 13 in]
                          n325 = call <vilib>:"Camera Get image.vi"("error in (no error)"=w772, "camera"=w773) -> ("error out"=w775:errorcluster, "Image"=w778:T12)  [unwired: 3 in, 1 out]
                          n326 = call "Image get data.vi"("error in (no error)"=w775, "Image Compat"=w778) -> ("error out"=w774:errorcluster, "Array"=w776:u32[][], "Image Compat (dup)"=w777:T12)  [unwired: 3 in]
                          n327 = local write "Camera image"(w776) -> ()
                          n328 = call <vilib>:"Simple Error Handler.vi"("type of dialog (OK msg:1)"=w782, "error in (no error)"=w783) -> ()  [unwired: 3 in, 5 out]
                        }
                        frame #2 {
                          n329 = call <vilib>:"Haso compute slopes.vi"("error in (no error)"=w802, "Image Compat"=w801, "Haso"=w800) -> ("error out"=w799:errorcluster, "Data Haso"=w798:T5)  [unwired: 1 in, 2 out]
                          n330 = call "DataHaso ctor copie.vi"("error in (no error)"=w799, "DataHaso"=w798) -> ("error out"=w797:errorcluster, "new DataHaso"=w796:T5)  [unwired: 3 in, 1 out]
                          n331 = Bundle By Name(cluster=T3 {"Filtre tilt X"=FALSE, "Filtre tilt Y"=FALSE, "Filtre courbure"=FALSE} ("Filtre"), "Filtre tilt X"="Filter x tilt 2", "Filtre tilt Y"="Filter y tilt 2", "Filtre courbure"="Curvature filter 2") -> (w806:T3)
                          n332 = call <vilib>:"DataHaso parameters.vi"("error in (no error)"=w797, "Data Haso"=w796) -> ("error out"=w812:errorcluster, "Parameters"=→"after correction":T1, "Data Haso (dup)"=w809:T5)  [unwired: 3 in]
                          n333 = call "DataHaso filter tilt or curvature.vi"("error in (no error)"=w812, "Filter (default: all true)"=w806, "Data Haso"=w809) -> ("error out"=w811:errorcluster, "Data Haso (dup)"=w808:T5)  [unwired: 3 in]
                          n334 = control-ref of="after correction"() -> (w813:refnum<vi>)
                          n335 = call "DataHaso phase.vi"("error in (no error)"=w811, "Data Haso"=w808) -> ("error out"=w814:errorcluster, "Phase (µm)"=w815:i32, "Data Haso (dup)"=w795:T5)  [unwired: 3 in]
                          n336 = call "Formatter Intensity Graph.vi"("error in (no error)"=w814, "Intensity Graph"=w813, "Surface with pupil"=w815) -> ("error out"=w793:errorcluster, "Surface with pupil (dup)"=w794:i32)  [unwired: 2 in, 1 out]
                          n337 = call <vilib>:"Surface with pupil get stats.vi"("error in (no error)"=w793, "Surface Avec Pupille"=w794) -> ("PV"=→"PV 2":sgl, "RMS"=→"RMS 2":dbl)  [unwired: 2 in, 2 out]
                        }
                        frame #3 {
                          n338 = flat-sequence {
                            tunnel: w818 -> [w820]
                            tunnel: w817 -> [w822]
                            tunnel: w816 -> [w821]
                            tunnel: w819 -> [w823]
                            frame #0 {
                              n339 = call "Casao dtor.vi"("Casao"=w820) -> ()  [unwired: 6 in, 1 out]
                            }
                            frame #1 {
                              n340 = call "DataHaso dtor.vi"("Data Haso"=w821) -> ()  [unwired: 6 in, 1 out]
                              n341 = call "DataHaso dtor.vi"("Data Haso"=w822) -> ()  [unwired: 6 in, 1 out]
                            }
                            frame #2 {
                              n342 = call "DataHaso dtor.vi"("Data Haso"=w823) -> ()  [unwired: 6 in, 1 out]
                            }
                          }
                        }
                      }
                    }
                    frame #4 {
                      w825 = T8 3 items=["no dialog", "OK message", "continue or stop message", "OK message + warnings", "continue/stop + warnings"] ("type of dialog (OK msg:1)")
                      w834 = T8 3 items=["no dialog", "OK message", "continue or stop message", "OK message + warnings", "continue/stop + warnings"] ("type of dialog (OK msg:1)")
                      n343 = call-poly <vilib>:"DAQmx Create Virtual Channel.vi"("lines"=tag "Dev1/port0/line2") -> ("task out"=w838:refnum<k21>, "error out"=w837:errorcluster)  [unwired: 13 in]
                      n344 = call-poly <vilib>:"DAQmx Create Virtual Channel.vi"("lines"=tag "Dev1/port0/line1") -> ("task out"=w829:refnum<k21>, "error out"=w828:errorcluster)  [unwired: 13 in]
                      n345 = call-poly <vilib>:"DAQmx Write.vi"("task/channels in"=w838, "auto start"=TRUE, "data"=FALSE ("Shutter"), "error in"=w837) -> ("task out"=w840:refnum<k21>, "error out"=w841:errorcluster)  [unwired: 9 in, 1 out]
                      n346 = call-poly <vilib>:"DAQmx Write.vi"("task/channels in"=w829, "auto start"=TRUE, "data"=FALSE ("Shutter"), "error in"=w828) -> ("task out"=w831:refnum<k21>, "error out"=w832:errorcluster)  [unwired: 9 in, 1 out]
                      n347 = call <vilib>:"DAQmx Clear Task.vi"("task in"=w840, "error in"=w841) -> ("error out"=w835:errorcluster)  [unwired: 13 in]
                      n348 = call <vilib>:"DAQmx Clear Task.vi"("task in"=w831, "error in"=w832) -> ("error out"=w826:errorcluster)  [unwired: 13 in]
                      n349 = call <vilib>:"Simple Error Handler.vi"("type of dialog (OK msg:1)"=w834, "error in (no error)"=w835) -> ()  [unwired: 3 in, 5 out]
                      n350 = call <vilib>:"Simple Error Handler.vi"("type of dialog (OK msg:1)"=w825, "error in (no error)"=w826) -> ()  [unwired: 3 in, 5 out]
                    }
                  }
                }
              }
            }
            frame #2 {
              w878 = 0.0  # Laser Power (%)
              w860 = 0.12  # Em Fast Galvo
              w842 = -0.12  # Em Slow Galvo
              w851 = 0.12  # Ex Slow Galvo
              w869 = 0.12  # Ex Fast Galvo
              w848 = T8 3 items=["no dialog", "OK message", "continue or stop message", "OK message + warnings", "continue/stop + warnings"] ("type of dialog (OK msg:1)")
              w857 = T8 3 items=["no dialog", "OK message", "continue or stop message", "OK message + warnings", "continue/stop + warnings"] ("type of dialog (OK msg:1)")
              w866 = T8 3 items=["no dialog", "OK message", "continue or stop message", "OK message + warnings", "continue/stop + warnings"] ("type of dialog (OK msg:1)")
              w875 = T8 3 items=["no dialog", "OK message", "continue or stop message", "OK message + warnings", "continue/stop + warnings"] ("type of dialog (OK msg:1)")
              w881 = T8 3 items=["no dialog", "OK message", "continue or stop message", "OK message + warnings", "continue/stop + warnings"] ("type of dialog (OK msg:1)")
              n351 = call-poly <vilib>:"DAQmx Create Virtual Channel.vi"("physical channels"=tag "Dev1/ao1") -> ("task out"=w853:refnum<k21>, "error out"=w852:errorcluster)  [unwired: 13 in]
              n352 = call-poly <vilib>:"DAQmx Create Virtual Channel.vi"("physical channels"=tag "Dev1/ao0") -> ("task out"=w871:refnum<k21>, "error out"=w870:errorcluster)  [unwired: 13 in]
              n353 = call-poly <vilib>:"DAQmx Create Virtual Channel.vi"("physical channels"=tag "Dev1/ao3") -> ("task out"=w844:refnum<k21>, "error out"=w843:errorcluster)  [unwired: 13 in]
              n354 = call-poly <vilib>:"DAQmx Create Virtual Channel.vi"("physical channels"=tag "Dev1/ao2") -> ("task out"=w862:refnum<k21>, "error out"=w861:errorcluster)  [unwired: 13 in]
              n355 = Multiply(x=w878, y=0.0137 ("data")) -> (x*y=w880:dbl)
              n356 = call-poly <vilib>:"DAQmx Create Virtual Channel.vi"("physical channels"=tag "Dev1/ao4") -> ("task out"=w887:refnum<k21>, "error out"=w888:errorcluster)  [unwired: 13 in]
              n357 = call-poly <vilib>:"DAQmx Write.vi"("task/channels in"=w853, "auto start"=TRUE, "data"=w851, "error in"=w852) -> ("task out"=w855:refnum<k21>, "error out"=w854:errorcluster)  [unwired: 9 in, 1 out]
              n358 = call-poly <vilib>:"DAQmx Write.vi"("task/channels in"=w871, "auto start"=TRUE, "data"=w869, "error in"=w870) -> ("task out"=w873:refnum<k21>, "error out"=w872:errorcluster)  [unwired: 9 in, 1 out]
              n359 = call-poly <vilib>:"DAQmx Write.vi"("task/channels in"=w844, "auto start"=TRUE, "data"=w842, "error in"=w843) -> ("task out"=w846:refnum<k21>, "error out"=w845:errorcluster)  [unwired: 9 in, 1 out]
              n360 = call-poly <vilib>:"DAQmx Write.vi"("task/channels in"=w862, "auto start"=TRUE, "data"=w860, "error in"=w861) -> ("task out"=w864:refnum<k21>, "error out"=w863:errorcluster)  [unwired: 9 in, 1 out]
              n361 = call <vilib>:"DAQmx Clear Task.vi"("task in"=w855, "error in"=w854) -> ("error out"=w856:errorcluster)  [unwired: 13 in]
              n362 = call <vilib>:"DAQmx Clear Task.vi"("task in"=w873, "error in"=w872) -> ("error out"=w874:errorcluster)  [unwired: 13 in]
              n363 = call <vilib>:"DAQmx Clear Task.vi"("task in"=w846, "error in"=w845) -> ("error out"=w847:errorcluster)  [unwired: 13 in]
              n364 = call <vilib>:"DAQmx Clear Task.vi"("task in"=w864, "error in"=w863) -> ("error out"=w865:errorcluster)  [unwired: 13 in]
              n365 = call-poly <vilib>:"DAQmx Write.vi"("task/channels in"=w887, "auto start"=TRUE, "data"=w880, "error in"=w888) -> ("task out"=w884:refnum<k21>, "error out"=w885:errorcluster)  [unwired: 9 in, 1 out]
              n366 = call <vilib>:"Simple Error Handler.vi"("type of dialog (OK msg:1)"=w857, "error in (no error)"=w856) -> ()  [unwired: 3 in, 5 out]
              n367 = call <vilib>:"Simple Error Handler.vi"("type of dialog (OK msg:1)"=w875, "error in (no error)"=w874) -> ()  [unwired: 3 in, 5 out]
              n368 = call <vilib>:"Simple Error Handler.vi"("type of dialog (OK msg:1)"=w848, "error in (no error)"=w847) -> ()  [unwired: 3 in, 5 out]
              n369 = call <vilib>:"Simple Error Handler.vi"("type of dialog (OK msg:1)"=w866, "error in (no error)"=w865) -> ()  [unwired: 3 in, 5 out]
              n370 = call <vilib>:"DAQmx Clear Task.vi"("task in"=w884, "error in"=w885) -> ("error out"=w882:errorcluster)  [unwired: 13 in]
              n371 = call <vilib>:"Simple Error Handler.vi"("type of dialog (OK msg:1)"=w881, "error in (no error)"=w882) -> ()  [unwired: 3 in, 5 out]
            }
          }
        }
      }
    }
  }
